vi "HEWH RLT Draw Tester.vi"(8 "Error In":errorcluster) -> (0 "Error Out":errorcluster)   [LabVIEW 2016]
uses:
  Utility/Type Definitions/UTILITY Notifier.ctl
  Utility/Save File/File Setup.lvlib
  Utility/Save File/File Setup (Public)/Type Definition/Save File DOE Configuration State.ctl
  Type Definitions/HEWH Valve Bank Positions.ctl
  Custom Instrument Control/MW100/Type Definitions/HEWH MW100 Channel Numbers.ctl
  Utility/LabVIEW GEA2 Toolkit v1.0.0.0/library/GEA2_Toolkit.lvlib
  Utility/Custom Pallet Controls/Custom Pallet DBL.ctl
  Type Definitions/HEWH Power Elements.ctl
  Type Definitions/HEWH Draw Pattern Setup.ctl
  Type Definitions/HEWH Termination Condition Cluster.ctl
  Type Definitions/HEWH Power Data.ctl
  Utility/Type Definitions/UTILITY Power Analyzer.ctl
  Type Definitions/HEWH Output Information.ctl
  Type Definitions/HEWH Tank Indicator.ctl
  Utility/Custom Pallet Controls/Custom Pallet Timer.ctl
  Type Definitions/HEWH RLT Cycle Conditions.ctl
  Utility/Type Definitions/UTILITY Power Inputs Control.ctl
  Drivers/IND560 Scale Monitor/Type Definitions/IND560 Configuration.ctl
  Type Definitions/HEWH Agilent Cluster.ctl
  Utility/Type Definitions/UTILITY TC Coefficients.ctl
  Washer DOE/Type Definitions/DOE Test Fixture Hardware.ctl
  Washer DOE/Configuration/GEA2.ctl
  Washer DOE/Type Definitions/DOE Capacity Measurments.ctl
  <vilib>/Platform/fileVersionInfo.llb/FileVersionInformation.ctl
  Utility/Custom Pallet Controls/Custom Pallet String.ctl
  Utility/Save File/File Setup (Public)/Type Definition/Save File DISH Dishwasher Details.ctl
  Washer DOE/Type Definitions/DOE Main Control.ctl
  Utility/Save File/File Setup (Public)/Type Definition/Save File DOE Data Save Filepaths.ctl
  Utility/Save File/File Setup (Public)/Type Definition/Save File DOE File Path Control.ctl
  Utility/Save File/File Setup (Public)/Type Definition/Save File DOE LabView Program.ctl
  Custom Instrument Control/MW100/Type Definitions/Station ID Selector.ctl
  Utility/Save File/File Setup (Public)/Type Definition/Save File HEWH Heating Control Mode.ctl
  Type Definitions/PRAT Test.ctl
  Type Definitions/HEWH Calc and Calibration.ctl
  Support VIs/Draw Water Specific/Type Definitions/Terminate Draw Conditions.ctl
  Type Definitions/HEWH Start Conditions.ctl
  Type Definitions/HEWH Specific DAQ.ctl
  Utility/Save File/Public/Type Definitions/Save File Unit Type.ctl
  Utility/Save File/Save File.lvlib
  Utility/Save File/Public/Type Definitions/Save File Appliance Display.ctl
  Utility/Save File/Public/Type Definitions/Save File Washer.ctl
  Support VIs/Draw Water Specific/Type Definitions/Check Special Condtions.ctl
  Type Definitions/HEWH Draw Flag ENUM.ctl
  Support VIs/Draw Water Specific/Type Definitions/HEWH Special Condition Check.ctl
  Drivers/Omega FMA-1600A Series Gas Flow Meter/Type Definitions/FMA1600A COM Ports.ctl
  Washer DOE/Type Definitions/DOE Appliance Common.ctl
  Washer DOE/Type Definitions/DOE Dryer Standard.ctl
  Utility/Save File/File Setup (Public)/Type Definition/DPT IMC Data.ctl
panel:
  out "Numeric":i32
  in  "Retry Count":i32=5
  out "MW100":refnum<visa-resource-name>
  out "Main Loop Rate":dbl format="%0.2f"
  out "File  Version":string="Parametric Stand"
  in  "Filepath Output":T1={"General Setup Paths"={"Calibration File Path"=path "C:/Program Files/GE/Washer DOE/CalibrationDates.txt", "DOE Capacity Path"=path "C:/Program Files/GE/Washer DOE/DOE Capacity.txt", "Data Folder Path"=path "C:/Program Files/GE/Washer DOE/CalibrationDates.txt", "RLT Backup Data Path"=path "C:/Program Files/GE/Washer DOE/CalibrationDates.txt", "Tool Base Path"=path "C:/Program Files/GE/Washer DOE/CalibrationDates.txt", "General Startup Config Path"=path "C:/Program Files/GE/Washer DOE/CalibrationDates.txt", "File Save Previous Run Path"=path "C:/Program Files/GE/Washer DOE/CalibrationDates.txt", "File Save Configuration Data Path"=path "C:/Program Files/GE/Washer DOE/CalibrationDates.txt"}, "Data File Paths"={"Data File Path"=path "", "Debug File Path"=path "", "Bus Log Path"=path "", "Current"=path "", "Summary"=path ""}, "New Summary Created"=FALSE, "Check Location Interval (Second)"=0}
  in  "Washer Controls":T3={"Test Fixture Hardware"={"Power "={"Yokogawa"={"WT210"={"Sample Rate (1: 0.25s)"=1, "A Range (12: 20A)"=12, "V Range (6: 600V)"=4, "Power VISA Yokogawa WT210"="WT210"}, "WT500"={"Power VISA Yokogawa WT500"="WT500", "V Range (8: 1000V)"=0, "I Range (7: 40A)"=0, "Update Rate (3: 500ms)"=2}, "WT310_2"={"Sample Rate (1: 0.25s)"=60, "A Range (12: 20A)"=11, "V Range (6: 600V)"=4, "Power VISA Yokogawa WT310_2"="WT310_2"}, "WT310_3"={"Sample Rate (1: 0.25s)"=1, "A Range (12: 20A)"=11, "V Range (6: 600V)"=4, "Power VISA Yokogawa WT310_3"="WT310_3"}}, "Aplus"={"Aplus IP Address"="192.168.1.101", "Remote Port"=502, "Instrument"="APLUS", "Instr Driver Revision"="1.03.0053"}, "Power Limits"={"Crest Factor"={"Upper Limit"=1.49, "Lower Limit"=1.34}, "Harmonic Content"={"Uthd"=2.0}, "Voltage"={"% Error"=2.0}, "Stability"={"<1 Watt "={"Wattage"=1.0, "Slope (mW/H)"=10.0}, ">1 Watt"={"1%Power/Hour"=1.0}}}, "Nominal Voltage"=120, "Time Limit (s)"=10800.0, "Power Variation Limit (%)"=50.0, "Power Supply"={"Chroma 61605"="CHROMA", "Use Chroma?"=FALSE}}, "Weight Scale"={"Com Options"={"IND560Scale VISA"="LaurelMeter_Hot", "IP Address"="192.168.1.50", "Remote Port"=502, "Setra Scale VISA"="SETRA", "GSE 350"="GSE350"}, "Select Scale"=""}, "Flow Rates"={"Laurel Cold IP Address"="", "Laurel Hot IP Address"="", "Hot Water Laurel VISA"="34972A_3", "Cold Water Laurel VISA"="MW100", "Remote Port"=0, "Laurel Communication Type"="", "Meters To Collect (Hot Cold)"="", "HOT Laurel Reference"=refnum, "COLD Laurel Reference"=refnum}, "Analog Data"={"Agilent"={"Agilent 34972_1"="34972A_1", "Agilent 34972_2"="34972A_2", "Agilent 34972_3"="34972A_3", "Agilent 34972_4"="34972A_3", "Agilent 34972_5"="34972A_3", "Agilent 34972_6"="34972A_3", "Agilent Gain"=0.0, "TC Type (K,J,T)"="", "Instrument IDN?"="", "TC Channels-List"="", "Analog Channels-List"="", "Agilent Cluster Array"=[], "TC Channels-List 2"="", "Analog Channels-List 2"=""}, "Yokogawa"={"MW100"="MW100", "Intellifaucet"=FALSE}, "Select Analog"="", "TC Coefficients"={"TC Coefficients 1"=[], "TC Coefficients 2"=[], "TC Coefficients 3"=[], "TC Coefficients 4"=[], "TC Coefficients 5"=[], "TC Coefficients 6"=[], "TC Coefficients 7"=[]}, "NI Tasks (Dryer DOE)"=["TC Temps-Module 1", "TC Temps-Module 2", "TC Temps-Module 3", "TC Temps-Module 4", "TC Temps-Module 5", "Gas and Temp-Module 6", "AC_DC Events-Module 7"], "Laurel Analog"={"Laurel IP (Water Temp)"="", "Laurel IP (Pressure)"=""}}, "ITHX-Temp Humidity"={"IP Address 1"="", "Remote Port"=0, "IP Address 2"="", "IP Address 3"=""}, "Gas Meter COM Ports"={"Gas Meter 1"="COM3", "Gas Meter 2"="COM4", "Gas Meter 3"="COM5", "Gas Meter 4"="COM6", "Gas Meter 5"="COM7", "Gas Meter 6"="COM8"}, "Barometric Pressure"={"HEISE 901A"="HEISE", "Use Barometer?"=FALSE}}, "GEA2"={"Address"=35, "Source"=228, "Viper/Hawk"=0}, "DOE Capacity Measurments"={"Weight 1"=35.0, "Model Number 1"="", "Temp 1"=0.0, "Serial Number 1"="", "Lab Number 1"="", "Lab Number 2"="", "Serial Number 2"="", "Temp 2"=0.0, "Model Number 2"="", "Weight 2"=0.0, "Lab Number 3"="", "Serial Number 3"="", "Temp 3"=0.0, "Model Number 3"="", "Weight 3"=0.0, "Lab Number 4"="", "Serial Number 4"="", "Temp 4"=0.0, "Model Number 4"="", "Weight 4"=0.0, "Capacity Measurment Output String"=[]}, "Initialize.Washer In"={"Appliance Details"={"FileVersionInfo"={"FileVersion"="", "ProductName"="", "InternalName"="", "CompanyName"="", "LegalCopyright"="", "FileDescription"=""}, "Dishwasher Info"={"Open Cup Weight (gm):"=0.0, "Auto Cup Weight (gm):"=0.0, "Detergent-Dish:"="", "Inlet Temperature-Dish:"="", "Cycle Mode-Dish:"="", "Unit Control-Dish:"="", "Manufacturer-Dish:"=""}, "Washer Info"={"Hot Water Temperature (Fahrenheit):"="", "Cold Water Temperature (Fahrenheit):"="", "Capacity (cu.ft):"=0.0, "Initial Cloth Weight:"=0.0, "Cloth Lot:"=60, "Model Family:"="", "Program Name:"="", "Cycle Selection:"="", "Wash Temperature:"="", "Rinse Temperature:"="", "Load Size:"=""}, "File Name Output Array"=[], "Calibration Output Array"=[], "Appliance Common"={"Engineer:"="", "Model Number:"="", "Serial Number:"="", "Comments:"="", "Station ID:"="", "Technician:"="", "TR Number:"="", "Lab ID:"="", "Voltage:"="", "Water Pressure (PSI):"="", "Test Date:"="", "Computer Name:"="", "IP Address:"="", "Ambient RH:"="", "Frequency:"="", "Build:"="", "Filename:"="", "Test Type:"="", "Load Run #:"=17, "Ambient Temperature (F):"="", "File Path:"=path "", "Cycles Per Year"=0}, "Water Heater"={"Heating Mode:"=""}, "Dryer"={"Heat Setting:"="", "Washer Water Temperature (60 ± 5°F):"=7, "Water Hardness (PPM):"=7, "Dryness Setting:"="", "Dryer Type:"="", "Exhaust:"="", "Drying Cycle:"="", "Load Type:"="", "Nominal Load Weight"="", "Dryer Initial IMC Data"={"Measured IMC (lbs)"=100.0, "Actual Initial RMC (%)"=7.0, "RMC (Desired %)"=5.0, "Bone Dry Wt(lbs)"=60.0, "Tolerance(%)"=5.0, "Actual Final RMC (%)"=7.0, "CEF (lbf/kWh)"=0.0, "Minimum Weight (lbf)"=0.0, "Average Weight (lbf)"=0.0, "Maximum Weight (lbf)"=0.0, "Measured IMC In Range?"=FALSE, "Moisture Reduction Factor"=55.5, "Field Use Factor"=1.04, "Empty Dryer Cold Weigth"=0.0, "Energy Standard"=enum."D2-Automatic Dryer", "Weight Cloth (lbs)"=0.0, "Relative Moisture Content (%)"=0.0, "Relative Moisture Content - Avg (%)"=0.0}}}, "Display Data (RLT)"={"Status Color"=0, "Serial Number Display"="", "Cycle Count Display"=0, "Station Label Display"="", "Current Run Start Time Display"=0.0, "Board ID Display"="", "RPM Display"=0, "Current Display"=0.0, "Current Path Display"=path "", "Saving Display"=FALSE, "Unit Type Display"=enum."", "Total Time On Display"=0.0, "UI Button"=FALSE}}} {"Initialize.Washer In"."Display Data (RLT)"."Current Display" format="%.2f"; "Initialize.Washer In"."Display Data (RLT)"."Cycle Count Display" format="%04d"; "Initialize.Washer In"."Appliance Details"."Dryer"."Dryer Initial IMC Data"."Maximum Weight (lbf)" format="%03_6g"; "Initialize.Washer In"."Appliance Details"."Dryer"."Dryer Initial IMC Data"."Average Weight (lbf)" format="%03_6g"; "Initialize.Washer In"."Appliance Details"."Dryer"."Dryer Initial IMC Data"."Minimum Weight (lbf)" format="%03_6g"; "Initialize.Washer In"."Appliance Details"."Dryer"."Dryer Initial IMC Data"."CEF (lbf/kWh)" format="%03_6g"; "Initialize.Washer In"."Appliance Details"."Dryer"."Dryer Initial IMC Data"."Actual Final RMC (%)" format="%03_6g"; "Initialize.Washer In"."Appliance Details"."Dryer"."Dryer Initial IMC Data"."Tolerance(%)" format="%0#_6g"; "Initialize.Washer In"."Appliance Details"."Dryer"."Dryer Initial IMC Data"."Bone Dry Wt(lbs)" format="%03_6g"; "Initialize.Washer In"."Appliance Details"."Dryer"."Dryer Initial IMC Data"."RMC (Desired %)" format="%0#_6g"; "Initialize.Washer In"."Appliance Details"."Dryer"."Dryer Initial IMC Data"."Actual Initial RMC (%)" format="%03_6g"; "Initialize.Washer In"."Appliance Details"."Dryer"."Dryer Initial IMC Data"."Measured IMC (lbs)" format="%0#_6g"; "GEA2"."Address" format="%x"; "GEA2"."Source" format="%x"; "GEA2"."Viper/Hawk" items=["Viper", "Hawk"]; "Test Fixture Hardware"."Power"."Yokogawa"."WT310_3"."V Range (6: 600V)" items=["Auto", "15V", "30V", "60V", "150V", "300V", "600V"]; "Test Fixture Hardware"."Power"."Yokogawa"."WT310_3"."A Range (12: 20A)" items=["Auto", "5mA", "10mA", "20mA", "50mA", "100mA", "200mA", "0.5A", "1A", "2A", "5A", "10A", "20A", "50mV", "100mV", "200mV", "2.5V", "5V", "10V"]; "Test Fixture Hardware"."Power"."Yokogawa"."WT310_3"."Sample Rate (1: 0.25s)" items=["0.1s", "0.25s", "0.5s", "1s", "2s", "5s"]; "Test Fixture Hardware"."Power"."Yokogawa"."WT310_2"."V Range (6: 600V)" items=["Auto", "15V", "30V", "60V", "150V", "300V", "600V"]; "Test Fixture Hardware"."Power"."Yokogawa"."WT310_2"."A Range (12: 20A)" items=["Auto", "5mA", "10mA", "20mA", "50mA", "100mA", "200mA", "0.5A", "1A", "2A", "5A", "10A", "20A", "50mV", "100mV", "200mV", "2.5V", "5V", "10V"]; "Test Fixture Hardware"."Power"."Yokogawa"."WT310_2"."Sample Rate (1: 0.25s)" items=["0.1s", "0.25s", "0.5s", "1s", "2s", "5s"]; "Test Fixture Hardware"."Power"."Yokogawa"."WT500"."Update Rate (3: 500ms)" items=["-", "100ms", "200ms", "500ms", "1s", "2s", "5s"]; "Test Fixture Hardware"."Power"."Yokogawa"."WT500"."I Range (7: 40A)" items=["AUTO", "500 mA", "1 A", "2 A", "5 A", "10 A", "20 A", "40 A", "S-AUTO", "50 mV", "100 mV", "200 mV", "500 mV", "1 V", "2 V", "5 V", "10 V", "250 mA", "500 mA", "1 A", "2.5 A", "5 A", "10 A", "20 A", "25 mV", "50 mV", "100 mV", "250 mV", "500 mV", "1 V", "2.5 V", "5 V"]; "Test Fixture Hardware"."Power"."Yokogawa"."WT500"."V Range (8: 1000V)" items=["AUTO", "15", "30", "60", "100", "150", "300", "600", "1000", "7.5", "15", "30", "50", "75", "150", "300", "500"]; "Test Fixture Hardware"."Power"."Yokogawa"."WT210"."V Range (6: 600V)" items=["Auto", "15V", "30V", "60V", "150V", "300V", "600V"]; "Test Fixture Hardware"."Power"."Yokogawa"."WT210"."A Range (12: 20A)" items=["Auto", "5mA", "10mA", "20mA", "50mA", "100mA", "200mA", "0.5A", "1A", "2A", "5A", "10A", "20A", "50mV", "100mV", "200mV", "2.5V", "5V", "10V"]; "Test Fixture Hardware"."Power"."Yokogawa"."WT210"."Sample Rate (1: 0.25s)" items=["0.1s", "0.25s", "0.5s", "1s", "2s", "5s"]}
  out "JKI Loop":i32
  out "Draw Loop":i32
  in  "Debug":bool
  out "States":string[](array[string])
  in  "Tab Control 2":enum32{"Setup", "Graph"}(tab)
  in  "Condition Cluster Output":T21={"Condition #1"=TRUE, "Condition #2"=FALSE, "Special Last Draw (HU Test)"=FALSE, "RTD Out Temperature <="=0.0, "Condition #3"=FALSE, "Mean Tank Temperature <="=0.0, "Condition #4"=FALSE, "Decrease Outlet Temperature \nBy (RTD Out)"=0.0, "Condition #5"=FALSE, "Condition #6"=FALSE, "Time (Seconds)"=0.0, "Condition #7"=FALSE, "Condition #8"=FALSE, "Draw Until Condition"={"UE"=FALSE, "LE"=FALSE, "COMP"=FALSE, "FANS"=FALSE}, "Condition #9"=FALSE}
  in  "Clear Graph Data":bool
  out "XY Graph":T23(graph)
  in  "Pause Graph":bool
  in  "X-Axis":string(combo)
  in  "Y-Axis-1":string(combo)
  in  "Y-Axis-2":string(combo)
  in  "HEWH Power":bool
  out "DAQ Data":T24={"HEWH Standard"={"Voltage (Volts)"=240.0, "Current (Amps)"=0.017575, "Power (Watts)"=4.218, "WattHours (Wh)"=19682.0, "TC Tree (AVG)"=0.0, "Flow Rate (GPM)"=0.0, "Gallons (Gal)"=0.0, "RTD Out (Deg F)"=0.0, "RTD In (Deg F)"=0.0, "RTD Amb (Deg F)"=0.0, "TC Down"=0.0, "UE Event Lead"=0, "LE Event Lead"=0, "TC Tree Array"=[]}, "PRAT"={"Power (Watts) A"=4192.0, "Power (Watts) B"=4192.0, "Power (Watts) C"=4192.0, "Power (Watts) D"=4192.0, "TC1"=0.0, "TC2"=0.0, "TC3"=0.0, "TC4"=0.0, "WattHours (Wh) A"=4192.0, "WattHours (Wh) B"=4192.0, "WattHours (Wh) C"=4192.0, "WattHours (Wh) D"=4192.0, "Ambient"=0.0, "Extra Temp"=0.0}, "Additional Power Data"={"Vthd"=236.2, "Frequency (Hz)"=236.2, "Apparent Power (VA)"=236.2, "Power Factor"=236.2, "Current Crest Factor"=236.2, "Voltage Crest Factor"=236.2, "Integration Time (sec)"=236.2}}
  out "Shutdown":bool=TRUE
  out "Delay Between Draws":T25 format="%<%H:%M:%S>t"
  out "Draw Complete":bool
  out "Timer Reset":bool
  out "Elapsed Time":T25 format="%<%H:%M:%S>t"
  in  "Tab Control":enum32{"Standard", "Custom"}(tab)
  out "Draw Count":i32
  in  "Cycle Condition":T26=enum."Time Delay (Seconds)"
  in  "Delay Between\nDraws (seconds)":dbl=60.0
  in  "Gallon Target":T27=6.0 format="%.2f"
  in  "Purge Time (Seconds)":T27=100.0 format="%.2f"
  in  "GPM Target":T27=3.0 format="%.2f"
  in  "Temperature":T27=58.0 format="%.2f"
  out "Set Status":T22
  out "MW100 Data":string[][](array[string])
  out "Tank Display":T28 {"TC6" format="%.2g"; "TIN" format="%.2g"; "TOUT" format="%.2g"; "TC5" format="%.2g"; "TC4" format="%.2g"; "TC3" format="%.2g"; "TC2" format="%.2g"; "TC1" format="%.2g"}
  in  "Reset Gallons":bool
  in  "Disable ERD A":bool
  in  "Use EMV List":bool=TRUE
  in  "Start UI Loop":bool=TRUE
  in  "Pressurize Tank":bool=TRUE
  in  "Stop Custom Draw":bool
  in  "Skip Draw":bool
  in  "Skip Purge":bool
  in  "Start Draw Override":bool
  in  "Start Test":bool
  out "Start Draw":bool
  out "Stop Draw Status":bool
  out "Pressurize Tank Status":bool
  out "UI Loop Status":bool
  out "Core HEWH Data out":T29={"Scan Rate Adjust"=0.0, "Draw Count"=0, "Test Patten Setup"={"Total Gallons Schedule"=[], "PRAT/RLT Sequence"=[{"Sequence #"=1.0, "Cycles"=35, "Mode Setting"="", "Flow Rate (GPM)"=0.0, "Temperature (F)"=0.0, "Reset Timer"=FALSE, "Use Temp Decline Method"=FALSE, "Terminate Condition"=enum."C1-Terminate Draw @ Gallon Mark", "Condition Value #1"=1.0, "UE"=FALSE, "LE"=FALSE, "Comp"=FALSE, "Fan"=FALSE, "Test End Time (Sec)"=0.0, "Purge Until Cutout"=FALSE, "Start Conditions"=enum."Heat Source Cutout", "Condition Value #2"=0.0, "Remove Power"=FALSE, "Time"=0.0, "Check Special Cond."=enum."SC1-Do Nothing", "Condition#"=enum."C1", "Draw Flags"=enum."N/A", "Data Processing Delay (FHD 15sec, UEF 5 Sec)"=0.0, "Test Complete"=FALSE}, {"Sequence #"=2.0, "Cycles"=15, "Mode Setting"="", "Flow Rate (GPM)"=0.0, "Temperature (F)"=0.0, "Reset Timer"=FALSE, "Use Temp Decline Method"=FALSE, "Terminate Condition"=enum."C1-Terminate Draw @ Gallon Mark", "Condition Value #1"=1.0, "UE"=FALSE, "LE"=FALSE, "Comp"=FALSE, "Fan"=FALSE, "Test End Time (Sec)"=0.0, "Purge Until Cutout"=FALSE, "Start Conditions"=enum."Heat Source Cutout", "Condition Value #2"=0.0, "Remove Power"=FALSE, "Time"=0.0, "Check Special Cond."=enum."SC1-Do Nothing", "Condition#"=enum."C1", "Draw Flags"=enum."N/A", "Data Processing Delay (FHD 15sec, UEF 5 Sec)"=0.0, "Test Complete"=FALSE}, {"Sequence #"=3.0, "Cycles"=35, "Mode Setting"="", "Flow Rate (GPM)"=0.0, "Temperature (F)"=0.0, "Reset Timer"=FALSE, "Use Temp Decline Method"=FALSE, "Terminate Condition"=enum."C1-Terminate Draw @ Gallon Mark", "Condition Value #1"=2.0, "UE"=FALSE, "LE"=FALSE, "Comp"=FALSE, "Fan"=FALSE, "Test End Time (Sec)"=0.0, "Purge Until Cutout"=FALSE, "Start Conditions"=enum."Heat Source Cutout", "Condition Value #2"=0.0, "Remove Power"=FALSE, "Time"=0.0, "Check Special Cond."=enum."SC1-Do Nothing", "Condition#"=enum."C1", "Draw Flags"=enum."N/A", "Data Processing Delay (FHD 15sec, UEF 5 Sec)"=0.0, "Test Complete"=FALSE}, {"Sequence #"=4.0, "Cycles"=15, "Mode Setting"="", "Flow Rate (GPM)"=0.0, "Temperature (F)"=0.0, "Reset Timer"=FALSE, "Use Temp Decline Method"=FALSE, "Terminate Condition"=enum."C1-Terminate Draw @ Gallon Mark", "Condition Value #1"=2.0, "UE"=FALSE, "LE"=FALSE, "Comp"=FALSE, "Fan"=FALSE, "Test End Time (Sec)"=0.0, "Purge Until Cutout"=FALSE, "Start Conditions"=enum."Heat Source Cutout", "Condition Value #2"=0.0, "Remove Power"=FALSE, "Time"=0.0, "Check Special Cond."=enum."SC1-Do Nothing", "Condition#"=enum."C1", "Draw Flags"=enum."N/A", "Data Processing Delay (FHD 15sec, UEF 5 Sec)"=0.0, "Test Complete"=FALSE}, {"Sequence #"=5.0, "Cycles"=35, "Mode Setting"="", "Flow Rate (GPM)"=0.0, "Temperature (F)"=0.0, "Reset Timer"=FALSE, "Use Temp Decline Method"=FALSE, "Terminate Condition"=enum."C1-Terminate Draw @ Gallon Mark", "Condition Value #1"=0.0, "UE"=FALSE, "LE"=FALSE, "Comp"=FALSE, "Fan"=FALSE, "Test End Time (Sec)"=0.0, "Purge Until Cutout"=FALSE, "Start Conditions"=enum."Heat Source Cutout", "Condition Value #2"=0.0, "Remove Power"=FALSE, "Time"=0.0, "Check Special Cond."=enum."SC1-Do Nothing", "Condition#"=enum."C1", "Draw Flags"=enum."N/A", "Data Processing Delay (FHD 15sec, UEF 5 Sec)"=0.0, "Test Complete"=FALSE}, {"Sequence #"=6.0, "Cycles"=15, "Mode Setting"="", "Flow Rate (GPM)"=0.0, "Temperature (F)"=0.0, "Reset Timer"=FALSE, "Use Temp Decline Method"=FALSE, "Terminate Condition"=enum."C1-Terminate Draw @ Gallon Mark", "Condition Value #1"=0.0, "UE"=FALSE, "LE"=FALSE, "Comp"=FALSE, "Fan"=FALSE, "Test End Time (Sec)"=0.0, "Purge Until Cutout"=FALSE, "Start Conditions"=enum."Heat Source Cutout", "Condition Value #2"=0.0, "Remove Power"=FALSE, "Time"=0.0, "Check Special Cond."=enum."SC1-Do Nothing", "Condition#"=enum."C1", "Draw Flags"=enum."N/A", "Data Processing Delay (FHD 15sec, UEF 5 Sec)"=0.0, "Test Complete"=FALSE}, {"Sequence #"=7.0, "Cycles"=35, "Mode Setting"="", "Flow Rate (GPM)"=0.0, "Temperature (F)"=0.0, "Reset Timer"=FALSE, "Use Temp Decline Method"=FALSE, "Terminate Condition"=enum."C1-Terminate Draw @ Gallon Mark", "Condition Value #1"=1.0, "UE"=FALSE, "LE"=FALSE, "Comp"=FALSE, "Fan"=FALSE, "Test End Time (Sec)"=0.0, "Purge Until Cutout"=FALSE, "Start Conditions"=enum."Heat Source Cutout", "Condition Value #2"=0.0, "Remove Power"=FALSE, "Time"=0.0, "Check Special Cond."=enum."SC1-Do Nothing", "Condition#"=enum."C1", "Draw Flags"=enum."N/A", "Data Processing Delay (FHD 15sec, UEF 5 Sec)"=0.0, "Test Complete"=FALSE}, {"Sequence #"=8.0, "Cycles"=15, "Mode Setting"="", "Flow Rate (GPM)"=0.0, "Temperature (F)"=0.0, "Reset Timer"=FALSE, "Use Temp Decline Method"=FALSE, "Terminate Condition"=enum."C1-Terminate Draw @ Gallon Mark", "Condition Value #1"=1.0, "UE"=FALSE, "LE"=FALSE, "Comp"=FALSE, "Fan"=FALSE, "Test End Time (Sec)"=0.0, "Purge Until Cutout"=FALSE, "Start Conditions"=enum."Heat Source Cutout", "Condition Value #2"=0.0, "Remove Power"=FALSE, "Time"=0.0, "Check Special Cond."=enum."SC1-Do Nothing", "Condition#"=enum."C1", "Draw Flags"=enum."N/A", "Data Processing Delay (FHD 15sec, UEF 5 Sec)"=0.0, "Test Complete"=FALSE}], "Current Sequence Index"=0}, "HEWH Specific DAQ"={"HEWH Data"={"HEWH Standard"={"Voltage (Volts)"=0.0, "Current (Amps)"=0.0, "Power (Watts)"=0.0, "WattHours (Wh)"=0.0, "TC Tree (AVG)"=0.0, "Flow Rate (GPM)"=0.0, "Gallons (Gal)"=0.0, "RTD Out (Deg F)"=0.0, "RTD In (Deg F)"=0.0, "RTD Amb (Deg F)"=0.0, "TC Down"=0.0, "UE Event Lead"=0, "LE Event Lead"=0, "TC Tree Array"=[]}, "PRAT"={"Power (Watts) A"=4192.0, "Power (Watts) B"=4192.0, "Power (Watts) C"=4192.0, "Power (Watts) D"=4192.0, "TC1"=0.0, "TC2"=0.0, "TC3"=0.0, "TC4"=0.0, "WattHours (Wh) A"=4192.0, "WattHours (Wh) B"=4192.0, "WattHours (Wh) C"=4192.0, "WattHours (Wh) D"=4192.0, "Ambient"=0.0, "Extra Temp"=0.0}, "Additional Power Data"={"Vthd"=236.2, "Frequency (Hz)"=236.2, "Apparent Power (VA)"=236.2, "Power Factor"=236.2, "Current Crest Factor"=236.2, "Voltage Crest Factor"=236.2, "Integration Time (sec)"=236.2}}, "Intellif Valve % Open"=0.0, "Power State"={"UE"=FALSE, "LE"=FALSE, "COMP"=FALSE, "FANS"=FALSE}, "Power Analyzer"=enum.""}, "Test Output Data"={"PreDraw Data Table"=[], "Data Table"=[], "MW100 TC Headers"=[]}, "Calc and Calibration"={"Mean SD Var Max Min Array"=[], "Draw Statistics (DBL)"=[], "Calibration Coefficients DBL"=[], "Start Gallons"=0.0, "Starting Temp Decline"=0.0, "K-Factor (Intellifaucet)"=0.0, "All Draw Stats"=[], "RTD Terminate Value"=0.0}, "Current Draw Time"=0.0, "LV Program"=enum."HEWH", "Station ID"=enum."A", "Current Cond"=enum."N/A", "Test Complete"=FALSE} {"Test Patten Setup"."PRAT/RLT Sequence"."Time" format="%<%H:%M:%S>t"; "Test Patten Setup"."Total Gallons Schedule" format="%.2f"}
  in  "Core HEWH Data Input":T29={"Scan Rate Adjust"=0.0, "Draw Count"=0, "Test Patten Setup"={"Total Gallons Schedule"=[], "PRAT/RLT Sequence"=[{"Sequence #"=1.0, "Cycles"=35, "Mode Setting"="", "Flow Rate (GPM)"=0.0, "Temperature (F)"=0.0, "Reset Timer"=FALSE, "Use Temp Decline Method"=FALSE, "Terminate Condition"=enum."C1-Terminate Draw @ Gallon Mark", "Condition Value #1"=1.0, "UE"=FALSE, "LE"=FALSE, "Comp"=FALSE, "Fan"=FALSE, "Test End Time (Sec)"=0.0, "Purge Until Cutout"=FALSE, "Start Conditions"=enum."Heat Source Cutout", "Condition Value #2"=0.0, "Remove Power"=FALSE, "Time"=0.0, "Check Special Cond."=enum."SC1-Do Nothing", "Condition#"=enum."C1", "Draw Flags"=enum."N/A", "Data Processing Delay (FHD 15sec, UEF 5 Sec)"=0.0, "Test Complete"=FALSE}, {"Sequence #"=2.0, "Cycles"=15, "Mode Setting"="", "Flow Rate (GPM)"=0.0, "Temperature (F)"=0.0, "Reset Timer"=FALSE, "Use Temp Decline Method"=FALSE, "Terminate Condition"=enum."C1-Terminate Draw @ Gallon Mark", "Condition Value #1"=1.0, "UE"=FALSE, "LE"=FALSE, "Comp"=FALSE, "Fan"=FALSE, "Test End Time (Sec)"=0.0, "Purge Until Cutout"=FALSE, "Start Conditions"=enum."Heat Source Cutout", "Condition Value #2"=0.0, "Remove Power"=FALSE, "Time"=0.0, "Check Special Cond."=enum."SC1-Do Nothing", "Condition#"=enum."C1", "Draw Flags"=enum."N/A", "Data Processing Delay (FHD 15sec, UEF 5 Sec)"=0.0, "Test Complete"=FALSE}, {"Sequence #"=3.0, "Cycles"=35, "Mode Setting"="", "Flow Rate (GPM)"=0.0, "Temperature (F)"=0.0, "Reset Timer"=FALSE, "Use Temp Decline Method"=FALSE, "Terminate Condition"=enum."C1-Terminate Draw @ Gallon Mark", "Condition Value #1"=2.0, "UE"=FALSE, "LE"=FALSE, "Comp"=FALSE, "Fan"=FALSE, "Test End Time (Sec)"=0.0, "Purge Until Cutout"=FALSE, "Start Conditions"=enum."Heat Source Cutout", "Condition Value #2"=0.0, "Remove Power"=FALSE, "Time"=0.0, "Check Special Cond."=enum."SC1-Do Nothing", "Condition#"=enum."C1", "Draw Flags"=enum."N/A", "Data Processing Delay (FHD 15sec, UEF 5 Sec)"=0.0, "Test Complete"=FALSE}, {"Sequence #"=4.0, "Cycles"=15, "Mode Setting"="", "Flow Rate (GPM)"=0.0, "Temperature (F)"=0.0, "Reset Timer"=FALSE, "Use Temp Decline Method"=FALSE, "Terminate Condition"=enum."C1-Terminate Draw @ Gallon Mark", "Condition Value #1"=2.0, "UE"=FALSE, "LE"=FALSE, "Comp"=FALSE, "Fan"=FALSE, "Test End Time (Sec)"=0.0, "Purge Until Cutout"=FALSE, "Start Conditions"=enum."Heat Source Cutout", "Condition Value #2"=0.0, "Remove Power"=FALSE, "Time"=0.0, "Check Special Cond."=enum."SC1-Do Nothing", "Condition#"=enum."C1", "Draw Flags"=enum."N/A", "Data Processing Delay (FHD 15sec, UEF 5 Sec)"=0.0, "Test Complete"=FALSE}, {"Sequence #"=5.0, "Cycles"=35, "Mode Setting"="", "Flow Rate (GPM)"=0.0, "Temperature (F)"=0.0, "Reset Timer"=FALSE, "Use Temp Decline Method"=FALSE, "Terminate Condition"=enum."C1-Terminate Draw @ Gallon Mark", "Condition Value #1"=0.0, "UE"=FALSE, "LE"=FALSE, "Comp"=FALSE, "Fan"=FALSE, "Test End Time (Sec)"=0.0, "Purge Until Cutout"=FALSE, "Start Conditions"=enum."Heat Source Cutout", "Condition Value #2"=0.0, "Remove Power"=FALSE, "Time"=0.0, "Check Special Cond."=enum."SC1-Do Nothing", "Condition#"=enum."C1", "Draw Flags"=enum."N/A", "Data Processing Delay (FHD 15sec, UEF 5 Sec)"=0.0, "Test Complete"=FALSE}, {"Sequence #"=6.0, "Cycles"=15, "Mode Setting"="", "Flow Rate (GPM)"=0.0, "Temperature (F)"=0.0, "Reset Timer"=FALSE, "Use Temp Decline Method"=FALSE, "Terminate Condition"=enum."C1-Terminate Draw @ Gallon Mark", "Condition Value #1"=0.0, "UE"=FALSE, "LE"=FALSE, "Comp"=FALSE, "Fan"=FALSE, "Test End Time (Sec)"=0.0, "Purge Until Cutout"=FALSE, "Start Conditions"=enum."Heat Source Cutout", "Condition Value #2"=0.0, "Remove Power"=FALSE, "Time"=0.0, "Check Special Cond."=enum."SC1-Do Nothing", "Condition#"=enum."C1", "Draw Flags"=enum."N/A", "Data Processing Delay (FHD 15sec, UEF 5 Sec)"=0.0, "Test Complete"=FALSE}, {"Sequence #"=7.0, "Cycles"=35, "Mode Setting"="", "Flow Rate (GPM)"=0.0, "Temperature (F)"=0.0, "Reset Timer"=FALSE, "Use Temp Decline Method"=FALSE, "Terminate Condition"=enum."C1-Terminate Draw @ Gallon Mark", "Condition Value #1"=1.0, "UE"=FALSE, "LE"=FALSE, "Comp"=FALSE, "Fan"=FALSE, "Test End Time (Sec)"=0.0, "Purge Until Cutout"=FALSE, "Start Conditions"=enum."Heat Source Cutout", "Condition Value #2"=0.0, "Remove Power"=FALSE, "Time"=0.0, "Check Special Cond."=enum."SC1-Do Nothing", "Condition#"=enum."C1", "Draw Flags"=enum."N/A", "Data Processing Delay (FHD 15sec, UEF 5 Sec)"=0.0, "Test Complete"=FALSE}, {"Sequence #"=8.0, "Cycles"=15, "Mode Setting"="", "Flow Rate (GPM)"=0.0, "Temperature (F)"=0.0, "Reset Timer"=FALSE, "Use Temp Decline Method"=FALSE, "Terminate Condition"=enum."C1-Terminate Draw @ Gallon Mark", "Condition Value #1"=1.0, "UE"=FALSE, "LE"=FALSE, "Comp"=FALSE, "Fan"=FALSE, "Test End Time (Sec)"=0.0, "Purge Until Cutout"=FALSE, "Start Conditions"=enum."Heat Source Cutout", "Condition Value #2"=0.0, "Remove Power"=FALSE, "Time"=0.0, "Check Special Cond."=enum."SC1-Do Nothing", "Condition#"=enum."C1", "Draw Flags"=enum."N/A", "Data Processing Delay (FHD 15sec, UEF 5 Sec)"=0.0, "Test Complete"=FALSE}], "Current Sequence Index"=0}, "HEWH Specific DAQ"={"HEWH Data"={"HEWH Standard"={"Voltage (Volts)"=0.0, "Current (Amps)"=0.0, "Power (Watts)"=0.0, "WattHours (Wh)"=0.0, "TC Tree (AVG)"=0.0, "Flow Rate (GPM)"=0.0, "Gallons (Gal)"=0.0, "RTD Out (Deg F)"=0.0, "RTD In (Deg F)"=0.0, "RTD Amb (Deg F)"=0.0, "TC Down"=0.0, "UE Event Lead"=0, "LE Event Lead"=0, "TC Tree Array"=[]}, "PRAT"={"Power (Watts) A"=4192.0, "Power (Watts) B"=4192.0, "Power (Watts) C"=4192.0, "Power (Watts) D"=4192.0, "TC1"=0.0, "TC2"=0.0, "TC3"=0.0, "TC4"=0.0, "WattHours (Wh) A"=4192.0, "WattHours (Wh) B"=4192.0, "WattHours (Wh) C"=4192.0, "WattHours (Wh) D"=4192.0, "Ambient"=0.0, "Extra Temp"=0.0}, "Additional Power Data"={"Vthd"=236.2, "Frequency (Hz)"=236.2, "Apparent Power (VA)"=236.2, "Power Factor"=236.2, "Current Crest Factor"=236.2, "Voltage Crest Factor"=236.2, "Integration Time (sec)"=236.2}}, "Intellif Valve % Open"=0.0, "Power State"={"UE"=FALSE, "LE"=FALSE, "COMP"=FALSE, "FANS"=FALSE}, "Power Analyzer"=enum.""}, "Test Output Data"={"PreDraw Data Table"=[], "Data Table"=[], "MW100 TC Headers"=[]}, "Calc and Calibration"={"Mean SD Var Max Min Array"=[], "Draw Statistics (DBL)"=[], "Calibration Coefficients DBL"=[], "Start Gallons"=0.0, "Starting Temp Decline"=0.0, "K-Factor (Intellifaucet)"=0.0, "All Draw Stats"=[], "RTD Terminate Value"=0.0}, "Current Draw Time"=0.0, "LV Program"=enum."HEWH", "Station ID"=enum."A", "Current Cond"=enum."N/A", "Test Complete"=FALSE} {"Test Patten Setup"."PRAT/RLT Sequence"."Time" format="%<%H:%M:%S>t"; "Test Patten Setup"."Total Gallons Schedule" format="%.2f"}
  out "Message":string="Purging and Calibrating Intellifaucet for 46 Seconds...."
  # "This was a bridge test software. Do not use"
  # "Select Only One Condition"
  # "Just Draw Water!"
  # "Condition #1"
  # "Draw Until Any Heat Source"
  # "Condition #2"
  # "Start Dispense Pattern"
  # "Draw Until Specific Heat Source"
  # "Condition #3"
  # "Dispense PRAT Sequence"
  # "Not Working"
  # "Condition #4"
  # "Condition #5"
  # "Condition #6"
  # "Next Cycle\nCondition"
  # "Conditions During Draw"
  # "Draw Pattern Setup (24 Hour)"
  # "Draw Pattern Setup (24 Hour)"
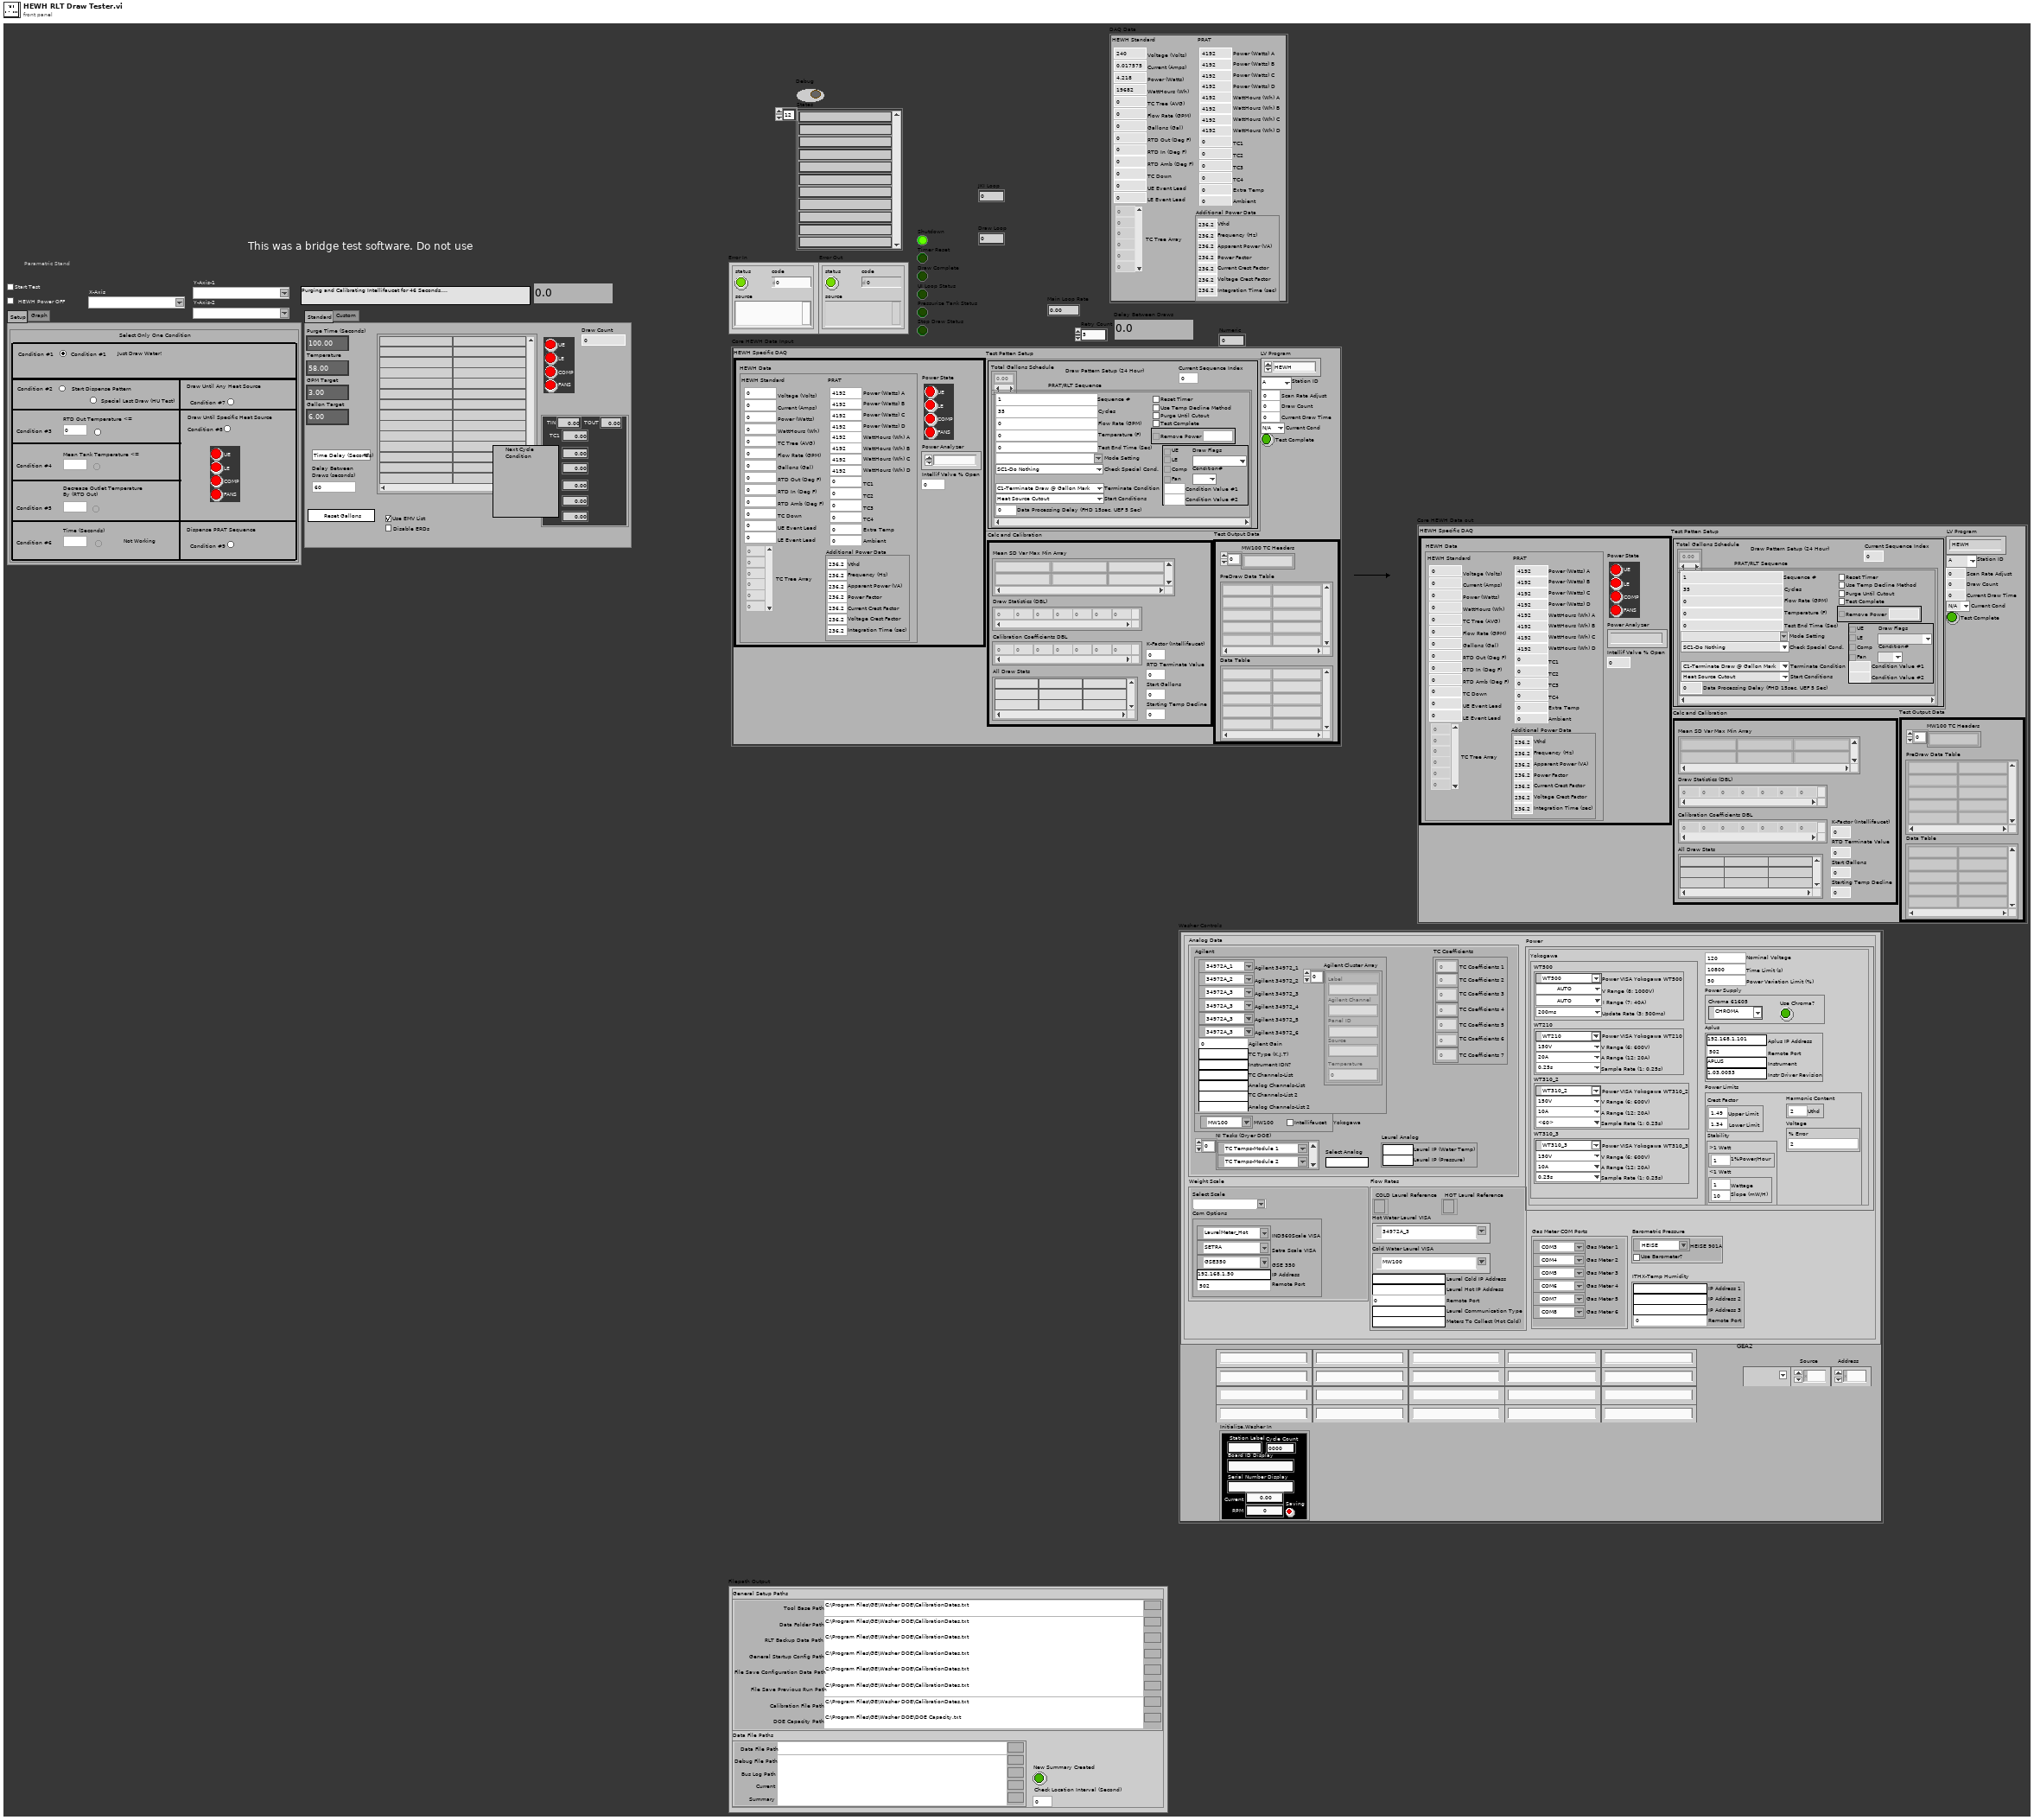
[diagram p1: front panel]
types:
  T1 = typedef "File Setup.lvlib/Save File DOE File Path Control.ctl" = cluster{"General Setup Paths":cluster{"Calibration File Path":path, "DOE Capacity Path":path, "Data Folder Path":path, "RLT Backup Data Path":path, "Tool Base Path":path, "General Startup Config Path":path, "File Save Previous Run Path":path, "File Save Configuration Data Path":path}, "Data File Paths":T2, "New Summary Created":bool, "Check Location Interval (Second)":i32}
  T2 = typedef "File Setup.lvlib/Save File DOE Data Save Filepaths.ctl" = cluster{"Data File Path":path, "Debug File Path":path, "Bus Log Path":path, "Current":path, "Summary":path}
  T3 = typedef "DOE Main Control.ctl" = cluster{"Test Fixture Hardware":T4, "GEA2":T10, "DOE Capacity Measurments":T11, "Initialize.Washer In":T12}
  T4 = typedef "DOE Test Fixture Hardware.ctl" = cluster{"Power ":T5, "Weight Scale":cluster{"Com Options":T6, "Select Scale":string}, "Flow Rates":cluster{"Laurel Cold IP Address":string, "Laurel Hot IP Address":string, "Hot Water Laurel VISA":refnum<visa-resource-name>, "Cold Water Laurel VISA":refnum<visa-resource-name>, "Remote Port":u16, "Laurel Communication Type":string, "Meters To Collect (Hot Cold)":string, "HOT Laurel Reference":refnum<k5>, "COLD Laurel Reference":refnum<k5>}, "Analog Data":cluster{"Agilent":cluster{"Agilent 34972_1":refnum<visa-resource-name>, "Agilent 34972_2":refnum<visa-resource-name>, "Agilent 34972_3":refnum<visa-resource-name>, "Agilent 34972_4":refnum<visa-resource-name>, "Agilent 34972_5":refnum<visa-resource-name>, "Agilent 34972_6":refnum<visa-resource-name>, "Agilent Gain":dbl, "TC Type (K,J,T)":string, "Instrument IDN?":string, "TC Channels-List":string, "Analog Channels-List":string, "Agilent Cluster Array":T7[], "TC Channels-List 2":string, "Analog Channels-List 2":string}, "Yokogawa":cluster{"MW100":refnum<visa-resource-name>, "Intellifaucet":bool}, "Select Analog":string, "TC Coefficients":T8, "NI Tasks (Dryer DOE)":refnum<k21>[], "Laurel Analog":cluster{"Laurel IP (Water Temp)":string, "Laurel IP (Pressure)":string}}, "ITHX-Temp Humidity":cluster{"IP Address 1":string, "Remote Port":u16, "IP Address 2":string, "IP Address 3":string}, "Gas Meter COM Ports":T9, "Barometric Pressure":cluster{"HEISE 901A":refnum<visa-resource-name>, "Use Barometer?":bool}}
  T5 = typedef "UTILITY Power Inputs Control.ctl" = cluster{"Yokogawa":cluster{"WT210":cluster{"Sample Rate (1: 0.25s)":i32, "A Range (12: 20A)":i32, "V Range (6: 600V)":i32, "Power VISA Yokogawa WT210":refnum<visa-resource-name>}, "WT500":cluster{"Power VISA Yokogawa WT500":refnum<visa-resource-name>, "V Range (8: 1000V)":i32, "I Range (7: 40A)":i32, "Update Rate (3: 500ms)":i32}, "WT310_2":cluster{"Sample Rate (1: 0.25s)":i32, "A Range (12: 20A)":i32, "V Range (6: 600V)":i32, "Power VISA Yokogawa WT310_2":refnum<visa-resource-name>}, "WT310_3":cluster{"Sample Rate (1: 0.25s)":i32, "A Range (12: 20A)":i32, "V Range (6: 600V)":i32, "Power VISA Yokogawa WT310_3":refnum<visa-resource-name>}}, "Aplus":cluster{"Aplus IP Address":string, "Remote Port":i32, "Instrument":string, "Instr Driver Revision":string}, "Power Limits":cluster{"Crest Factor":cluster{"Upper Limit":dbl, "Lower Limit":dbl}, "Harmonic Content":cluster{"Uthd":dbl}, "Voltage":cluster{"% Error":dbl}, "Stability":cluster{"<1 Watt ":cluster{"Wattage":dbl, "Slope (mW/H)":dbl}, ">1 Watt":cluster{"1%Power/Hour":dbl}}}, "Nominal Voltage":i32, "Time Limit (s)":dbl, "Power Variation Limit (%)":dbl, "Power Supply":cluster{"Chroma 61605":refnum<visa-resource-name>, "Use Chroma?":bool}}
  T6 = typedef "IND560 Configuration.ctl" = cluster{"IND560Scale VISA":refnum<visa-resource-name>, "IP Address":string, "Remote Port":u16, "Setra Scale VISA":refnum<visa-resource-name>, "GSE 350":refnum<visa-resource-name>}
  T7 = typedef "HEWH Agilent Cluster.ctl" = cluster{"Label":string, "Agilent Channel":string, "Panel ID":string, "Source":string, "Temperature":dbl}
  T8 = typedef "UTILITY TC Coefficients.ctl" = cluster{"TC Coefficients 1":dbl[], "TC Coefficients 2":dbl[], "TC Coefficients 3":dbl[], "TC Coefficients 4":dbl[], "TC Coefficients 5":dbl[], "TC Coefficients 6":dbl[], "TC Coefficients 7":dbl[]}
  T9 = typedef "FMA1600A COM Ports.ctl" = cluster{"Gas Meter 1":refnum<visa-resource-name>, "Gas Meter 2":refnum<visa-resource-name>, "Gas Meter 3":refnum<visa-resource-name>, "Gas Meter 4":refnum<visa-resource-name>, "Gas Meter 5":refnum<visa-resource-name>, "Gas Meter 6":refnum<visa-resource-name>}
  T10 = typedef "GEA2.ctl" = cluster{"Address":u8, "Source":u8, "Viper/Hawk":u8}
  T11 = typedef "DOE Capacity Measurments.ctl" = cluster{"Weight 1":dbl, "Model Number 1":string, "Temp 1":dbl, "Serial Number 1":string, "Lab Number 1":string, "Lab Number 2":string, "Serial Number 2":string, "Temp 2":dbl, "Model Number 2":string, "Weight 2":dbl, "Lab Number 3":string, "Serial Number 3":string, "Temp 3":dbl, "Model Number 3":string, "Weight 3":dbl, "Lab Number 4":string, "Serial Number 4":string, "Temp 4":dbl, "Model Number 4":string, "Weight 4":dbl, "Capacity Measurment Output String":string[][]}
  T12 = typedef "Save File.lvlib/Save File Washer.ctl" = cluster{"Appliance Details":T13, "Display Data (RLT)":T19}
  T13 = typedef "File Setup.lvlib/Save File DISH Dishwasher Details.ctl" = cluster{"FileVersionInfo":T14, "Dishwasher Info":cluster{"Open Cup Weight (gm):":dbl, "Auto Cup Weight (gm):":dbl, "Detergent-Dish:":string, "Inlet Temperature-Dish:":string, "Cycle Mode-Dish:":string, "Unit Control-Dish:":string, "Manufacturer-Dish:":string}, "Washer Info":cluster{"Hot Water Temperature (Fahrenheit):":string, "Cold Water Temperature (Fahrenheit):":string, "Capacity (cu.ft):":dbl, "Initial Cloth Weight:":dbl, "Cloth Lot:":i32, "Model Family:":string, "Program Name:":string, "Cycle Selection:":string, "Wash Temperature:":string, "Rinse Temperature:":string, "Load Size:":string}, "File Name Output Array":string[][], "Calibration Output Array":string[][], "Appliance Common":T15, "Water Heater":cluster{"Heating Mode:":string}, "Dryer":cluster{"Heat Setting:":T16, "Washer Water Temperature (60 ± 5°F):":u16, "Water Hardness (PPM):":u16, "Dryness Setting:":T16, "Dryer Type:":string, "Exhaust:":string, "Drying Cycle:":string, "Load Type:":string, "Nominal Load Weight":string, "Dryer Initial IMC Data":T17}}
  T14 = typedef "FileVersionInformation.ctl" = cluster{"FileVersion":string, "ProductName":string, "InternalName":string, "CompanyName":string, "LegalCopyright":string, "FileDescription":string}
  T15 = typedef "DOE Appliance Common.ctl" = cluster{"Engineer:":string, "Model Number:":string, "Serial Number:":string, "Comments:":string, "Station ID:":string, "Technician:":string, "TR Number:":string, "Lab ID:":string, "Voltage:":string, "Water Pressure (PSI):":string, "Test Date:":string, "Computer Name:":string, "IP Address:":string, "Ambient RH:":string, "Frequency:":string, "Build:":string, "Filename:":string, "Test Type:":string, "Load Run #:":i32, "Ambient Temperature (F):":string, "File Path:":path, "Cycles Per Year":u32}
  T16 = typedef "Custom Pallet String.ctl" = string
  T17 = typedef "DPT IMC Data.ctl" = cluster{"Measured IMC (lbs)":dbl, "Actual Initial RMC (%)":dbl, "RMC (Desired %)":dbl, "Bone Dry Wt(lbs)":dbl, "Tolerance(%)":dbl, "Actual Final RMC (%)":dbl, "CEF (lbf/kWh)":dbl, "Minimum Weight (lbf)":dbl, "Average Weight (lbf)":dbl, "Maximum Weight (lbf)":dbl, "Measured IMC In Range?":bool, "Moisture Reduction Factor":dbl, "Field Use Factor":dbl, "Empty Dryer Cold Weigth":dbl, "Energy Standard":T18, "Weight Cloth (lbs)":dbl, "Relative Moisture Content (%)":dbl, "Relative Moisture Content - Avg (%)":dbl}
  T18 = typedef "DOE Dryer Standard.ctl" = enum16{"D2-Automatic Dryer", "D2-Timer Dryer", "D1-Automatic Dryer", "D1-Timer Dryer", "Other"}
  T19 = typedef "Save File Appliance Display.ctl" = cluster{"Status Color":u32, "Serial Number Display":string, "Cycle Count Display":i32, "Station Label Display":string, "Current Run Start Time Display":dbl, "Board ID Display":string, "RPM Display":u32, "Current Display":dbl, "Current Path Display":path, "Saving Display":bool, "Unit Type Display":T20, "Total Time On Display":dbl, "UI Button":bool}
  T20 = typedef "Save File.lvlib/Save File Unit Type.ctl" = enum32{"", "Viper", "Hawk", "2015"}
  T21 = typedef "HEWH Termination Condition Cluster.ctl" = cluster{"Condition #1":bool, "Condition #2":bool, "Special Last Draw (HU Test)":bool, "RTD Out Temperature <=":dbl, "Condition #3":bool, "Mean Tank Temperature <=":dbl, "Condition #4":bool, "Decrease Outlet Temperature \nBy (RTD Out)":dbl, "Condition #5":bool, "Condition #6":bool, "Time (Seconds)":dbl, "Condition #7":bool, "Condition #8":bool, "Draw Until Condition":T22, "Condition #9":bool}
  T22 = typedef "HEWH Power Elements.ctl" = cluster{"UE":bool, "LE":bool, "COMP":bool, "FANS":bool}
  T23 = cluster{"Time Array Output":dbl[], "Data Array Output":dbl[]}[]
  T24 = typedef "HEWH Power Data.ctl" = cluster{"HEWH Standard":cluster{"Voltage (Volts)":dbl, "Current (Amps)":dbl, "Power (Watts)":dbl, "WattHours (Wh)":dbl, "TC Tree (AVG)":dbl, "Flow Rate (GPM)":dbl, "Gallons (Gal)":dbl, "RTD Out (Deg F)":dbl, "RTD In (Deg F)":dbl, "RTD Amb (Deg F)":dbl, "TC Down":dbl, "UE Event Lead":i32, "LE Event Lead":i32, "TC Tree Array":dbl[]}, "PRAT":cluster{"Power (Watts) A":dbl, "Power (Watts) B":dbl, "Power (Watts) C":dbl, "Power (Watts) D":dbl, "TC1":dbl, "TC2":dbl, "TC3":dbl, "TC4":dbl, "WattHours (Wh) A":dbl, "WattHours (Wh) B":dbl, "WattHours (Wh) C":dbl, "WattHours (Wh) D":dbl, "Ambient":dbl, "Extra Temp":dbl}, "Additional Power Data":cluster{"Vthd":dbl, "Frequency (Hz)":dbl, "Apparent Power (VA)":dbl, "Power Factor":dbl, "Current Crest Factor":dbl, "Voltage Crest Factor":dbl, "Integration Time (sec)":dbl}}
  T25 = typedef "Custom Pallet Timer.ctl" = dbl
  T26 = typedef "HEWH RLT Cycle Conditions.ctl" = enum16{"Manual", "Full Cutout", "Time Delay (Seconds)"}
  T27 = typedef "Custom Pallet DBL.ctl" = dbl
  T28 = typedef "HEWH Tank Indicator.ctl" = cluster{"TC1":dbl, "TC2":dbl, "TC3":dbl, "TC4":dbl, "TC5":dbl, "TIN":dbl, "TOUT":dbl, "TC6":dbl, "TC6-Color":u32, "TC5-Color":u32, "TC4-Color":u32, "TC3-Color":u32, "TC2-Color":u32, "TC1-Color":u32, "RTD-Out":u32, "RTD-In":u32}
  T29 = typedef "HEWH Output Information.ctl" = cluster{"Scan Rate Adjust":dbl, "Draw Count":i32, "Test Patten Setup":T30, "HEWH Specific DAQ":T38, "Test Output Data":cluster{"PreDraw Data Table":string[][], "Data Table":string[][], "MW100 TC Headers":string[]}, "Calc and Calibration":T40, "Current Draw Time":dbl, "LV Program":T41, "Station ID":T42, "Current Cond":T36, "Test Complete":bool}
  T30 = typedef "HEWH Draw Pattern Setup.ctl" = cluster{"Total Gallons Schedule":dbl[], "PRAT/RLT Sequence":T31[], "Current Sequence Index":i32}
  T31 = typedef "PRAT Test.ctl" = cluster{"Sequence #":dbl, "Cycles":i32, "Mode Setting":T32, "Flow Rate (GPM)":dbl, "Temperature (F)":dbl, "Reset Timer":bool, "Use Temp Decline Method":bool, "Terminate Condition":T33, "Condition Value #1":dbl, "UE":bool, "LE":bool, "Comp":bool, "Fan":bool, "Test End Time (Sec)":dbl, "Purge Until Cutout":bool, "Start Conditions":T34, "Condition Value #2":dbl, "Remove Power":bool, "Time":dbl, "Check Special Cond.":T35, "Condition#":T36, "Draw Flags":T37, "Data Processing Delay (FHD 15sec, UEF 5 Sec)":dbl, "Test Complete":bool}
  T32 = typedef "File Setup.lvlib/Save File HEWH Heating Control Mode.ctl" = string
  T33 = typedef "Terminate Draw Conditions.ctl" = enum16{"C1-Terminate Draw @ Gallon Mark", "C2-Special Last Draw (HU Test)", "C3-RTD Out <=", "C4-Mean Tank Temp <=", "C5-Decrease RTD Out (Deg F)", "C6-Time (Seconds)", "C7-Until Any Heat Source", "C8-Specific Heat Source", "C9-Do Nothing"}
  T34 = typedef "HEWH Start Conditions.ctl" = enum16{"Heat Source Cutout", "At Time (Seconds)", "Every X (Seconds)", "T2 >= X° Below Setpoint", "Seconds From Complete", "Wait for LE & Comp Cutout", "Wait for Comp Cutout", "Wait for LE Cutout", "Wait for UE Cutout"}
  T35 = typedef "Check Special Condtions.ctl" = enum16{"SC1-Do Nothing", "SC2-Check Heat Source (On-C2/Off-C1)", "SC3-Check Skip Condition", "SC4-Check Heat Source ON/Fail"}
  T36 = typedef "HEWH Special Condition Check.ctl" = enum16{"N/A", "C1", "C2", "Reset/Fail", "Skip Draw Sequence"}
  T37 = typedef "HEWH Draw Flag ENUM.ctl" = enum16{"N/A", "None(0)", "Sml(1)", "Med(2)", "SmlMed(3)", "Lrg(4)", "SmlLrg(5)", "MedLrg(6)", "SmlMedLrg(7)"}
  T38 = typedef "HEWH Specific DAQ.ctl" = cluster{"HEWH Data":T24, "Intellif Valve % Open":dbl, "Power State":T22, "Power Analyzer":T39}
  T39 = typedef "UTILITY Power Analyzer.ctl" = enum16{"", "APLUS", "WT210", "WT500", "WT300", "OSI", "Debug", "WT230", "WT300_1", "WT300_2"}
  T40 = typedef "HEWH Calc and Calibration.ctl" = cluster{"Mean SD Var Max Min Array":string[][], "Draw Statistics (DBL)":dbl[][], "Calibration Coefficients DBL":dbl[][], "Start Gallons":dbl, "Starting Temp Decline":dbl, "K-Factor (Intellifaucet)":dbl, "All Draw Stats":string[][], "RTD Terminate Value":dbl}
  T41 = typedef "File Setup.lvlib/Save File DOE LabView Program.ctl" = enum16{"No Name Found", "DOE Stand", "Dishwasher Kitchen", "Portable Stand", "HEWH", "Dryer", "Dryer WILT", "HCC", "PRAT", "HEWH RLT"}
  T42 = typedef "Station ID Selector.ctl" = enum16{"", "A", "B", "C", "D", "Global"}
  T43 = typedef "Semaphore RefNum" = refnum<k1>
  T44 = enum32{"invalid app kind", "Development System", "Run Time System", "Student Edition", "Embedded LabVIEW", "Evaluation", "Custom"}
  T45 = typedef "UTILITY Notifier.ctl" = enum16{"Set", "Read", "Release Ref"}
  T46 = typedef "HEWH Valve Bank Positions.ctl" = enum16{"Heating", "Purge", "Resting", "Draw"}
  T47 = enum32{"Invalid", "Standard", "Closed", "Hidden", "Minimized", "Maximized"}
  T48 = typedef "File Setup.lvlib/Save File DOE Configuration State.ctl" = enum16{"Open Front Panel", "Load Config"}
  T49 = typedef "HEWH MW100 Channel Numbers.ctl" = string
  T50 = cluster{"Core":cluster{"Current VI Reference":refnum<vi>, "Close Panel on Exit?":bool}, "Washer Controls":T3, "Filepath Output":T1, "Core HEWH Data Input":T29, "Main Power":bool, "Plot Array":dbl[][], "Total Array":string[][], "Save Data":string[][]}
  T51 = cluster{"Current VI Reference":refnum<vi>, "Close Panel on Exit?":bool}
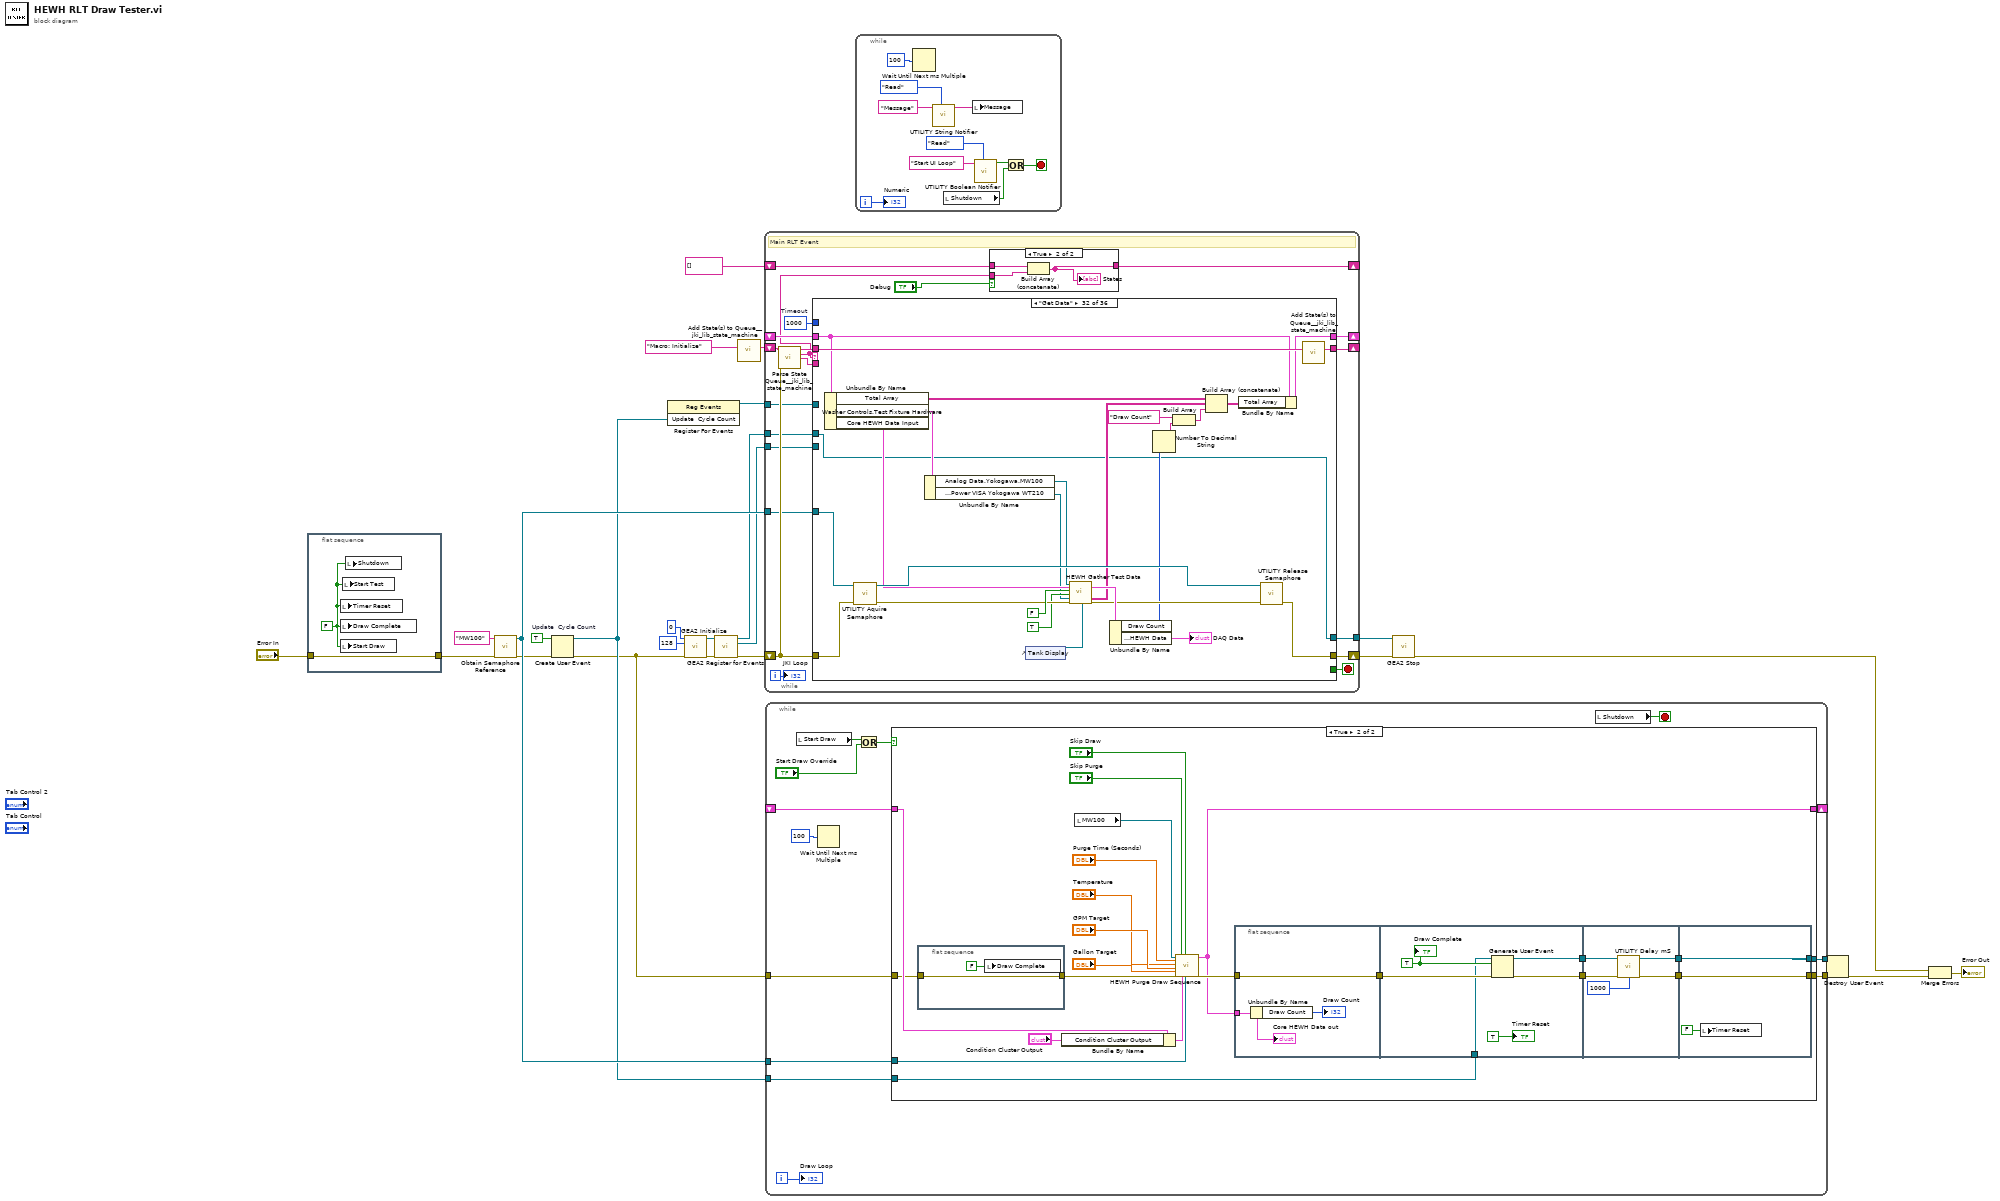
[diagram p0: block diagram]
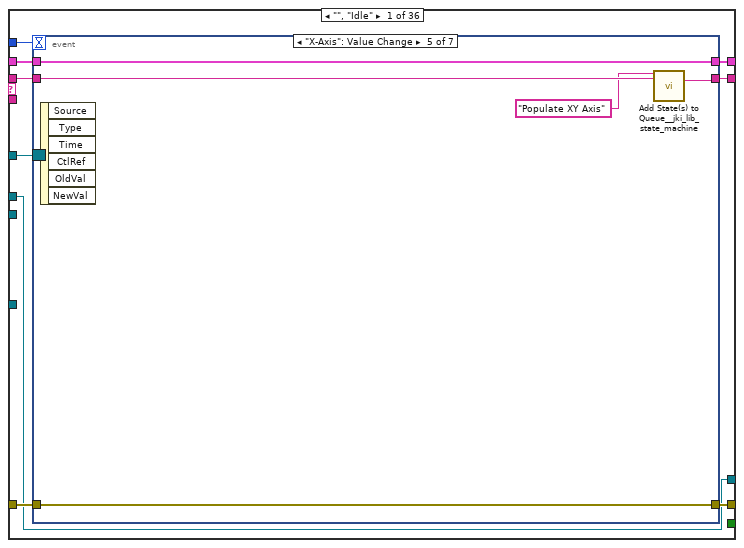
[diagram p3: hidden frame]
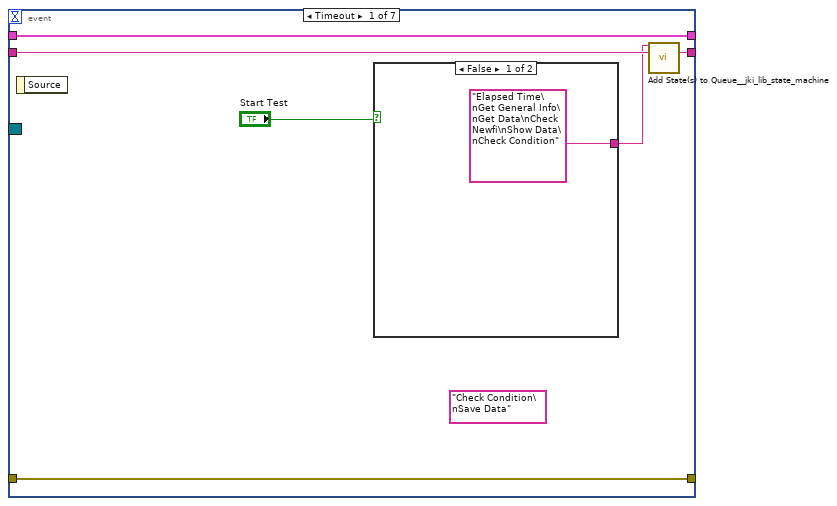
[diagram p4: hidden frame]
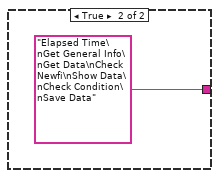
[diagram p5: hidden frame]
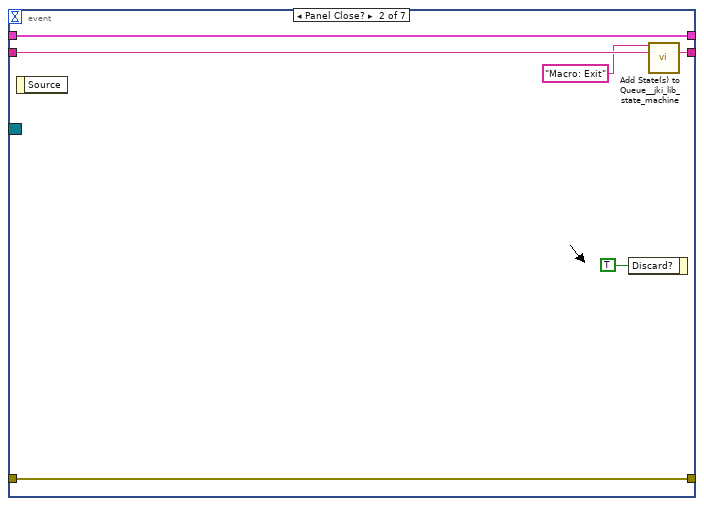
[diagram p6: hidden frame]
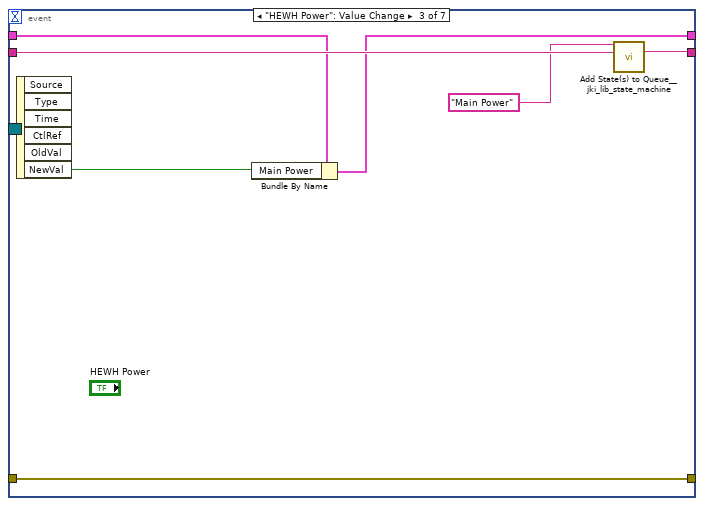
[diagram p7: hidden frame]
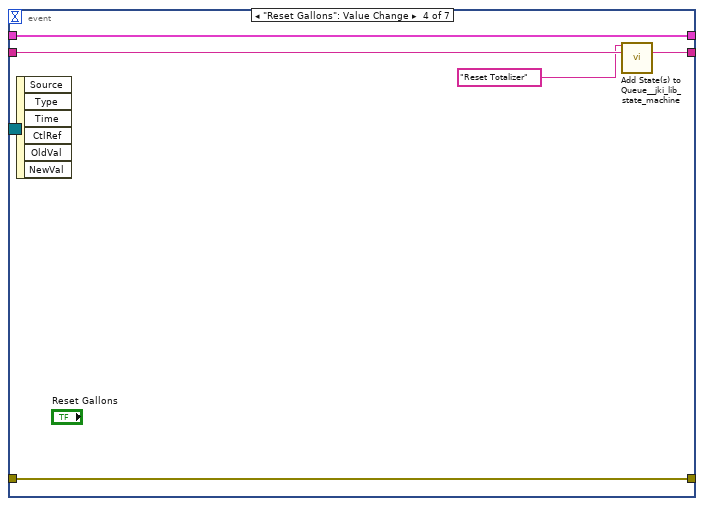
[diagram p8: hidden frame]
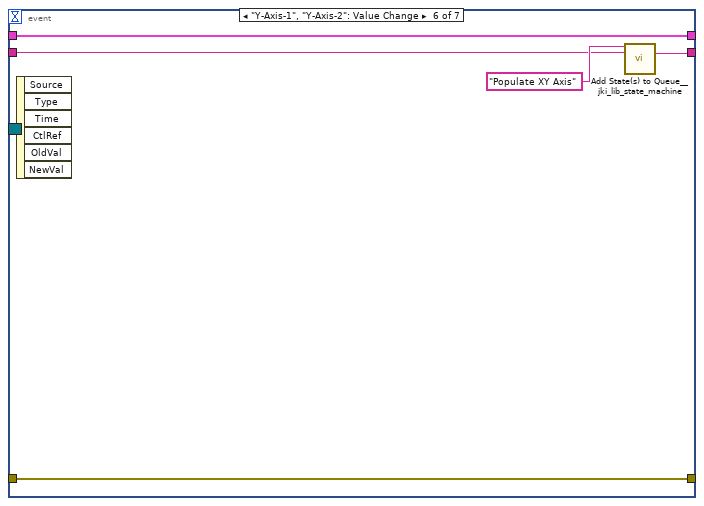
[diagram p9: hidden frame]
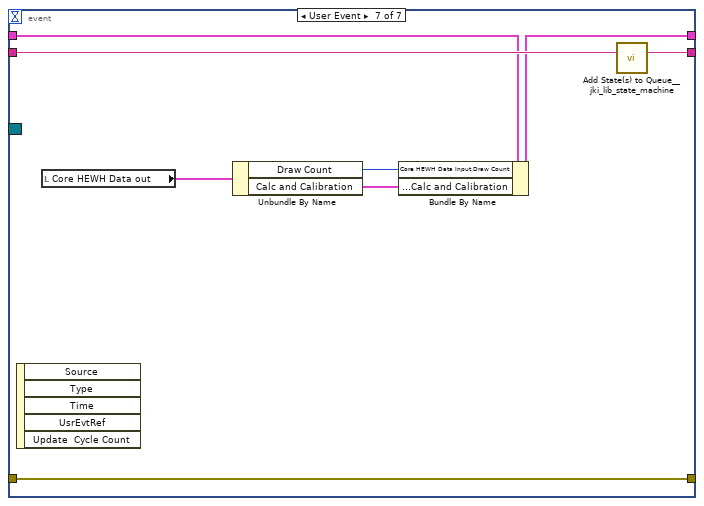
[diagram p10: hidden frame]
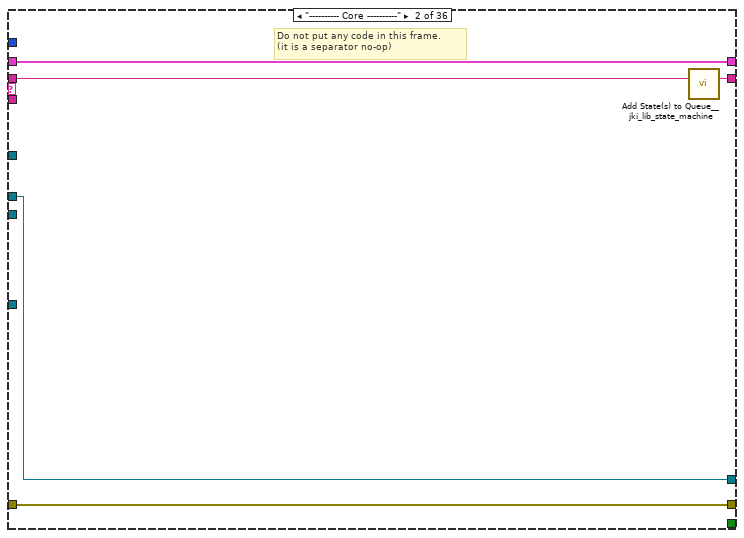
[diagram p11: hidden frame]
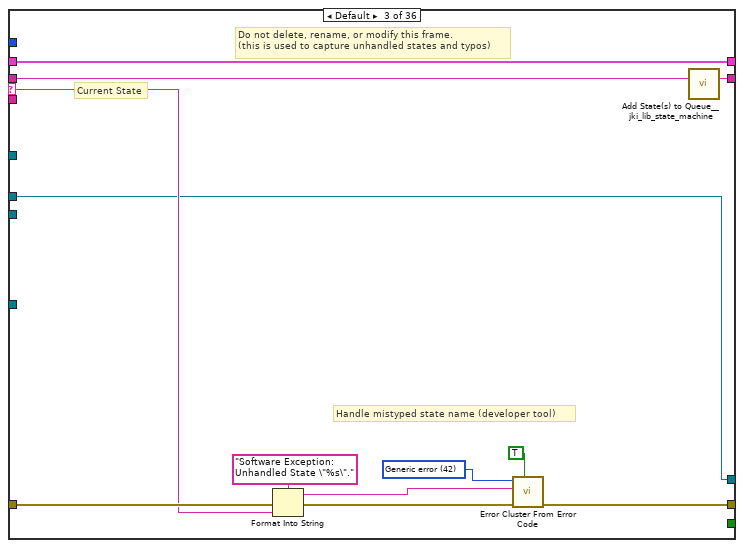
[diagram p12: hidden frame]
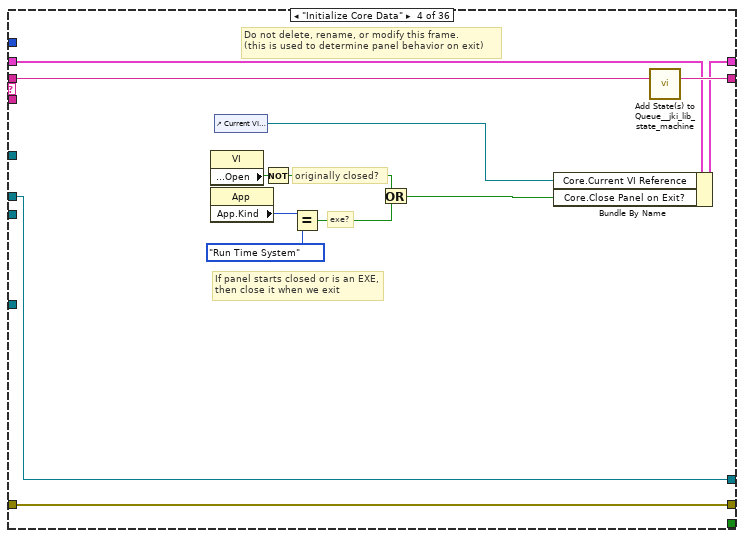
[diagram p13: hidden frame]
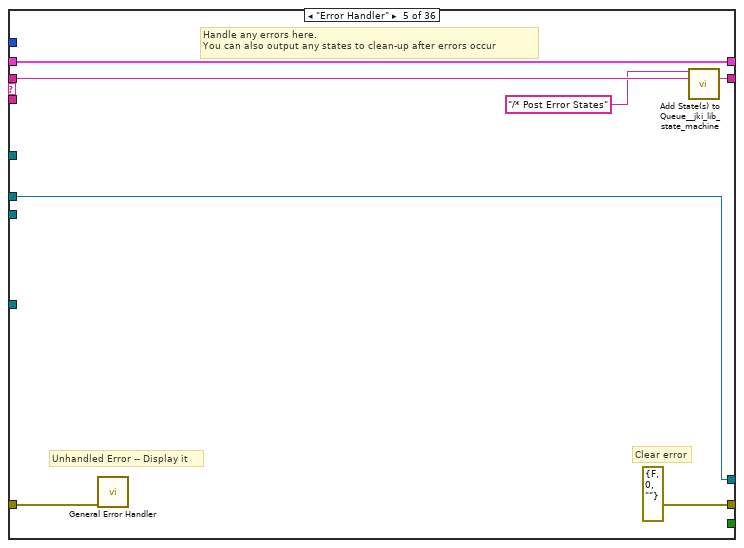
[diagram p14: hidden frame]
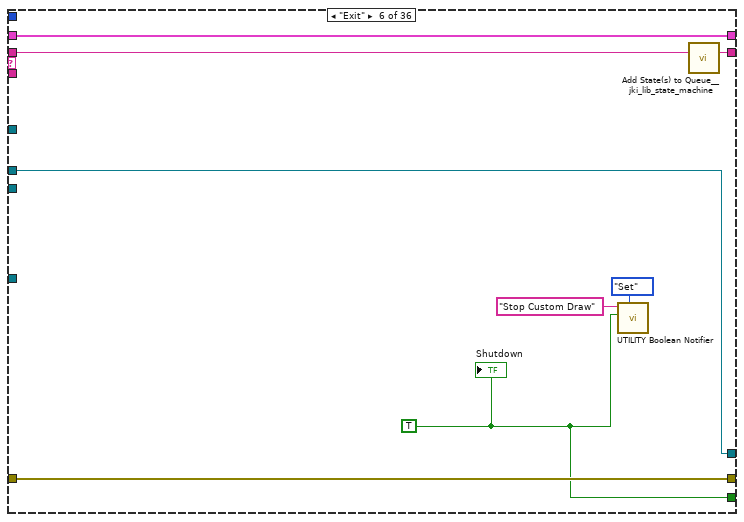
[diagram p15: hidden frame]
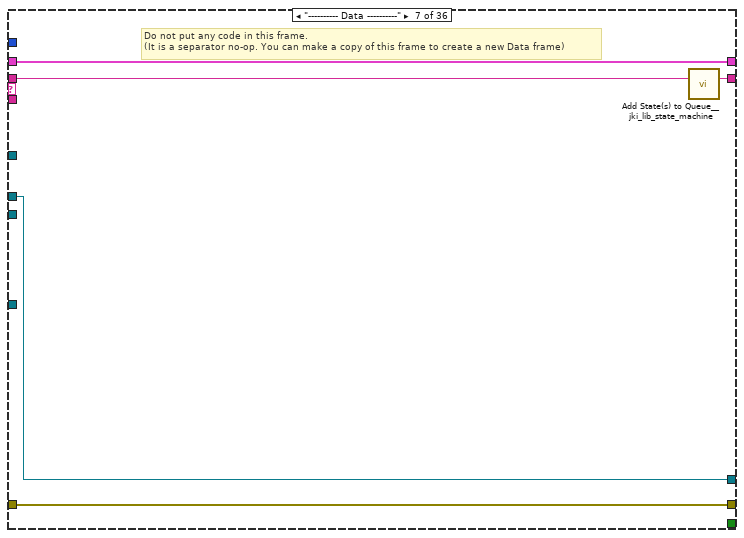
[diagram p16: hidden frame]
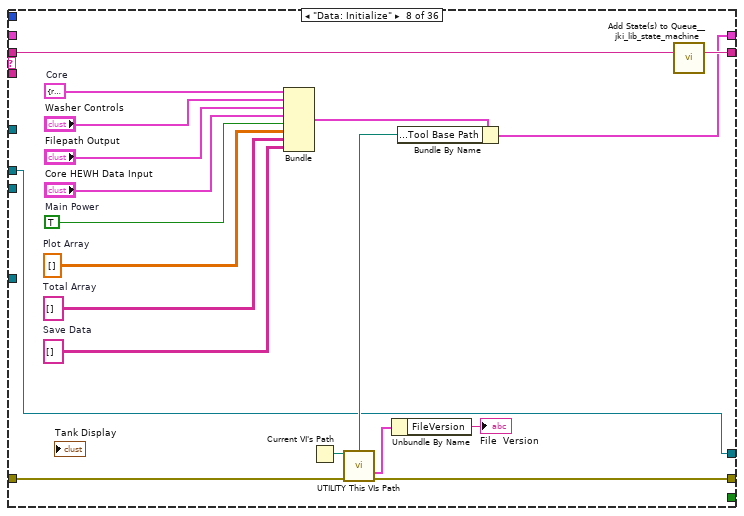
[diagram p17: hidden frame]
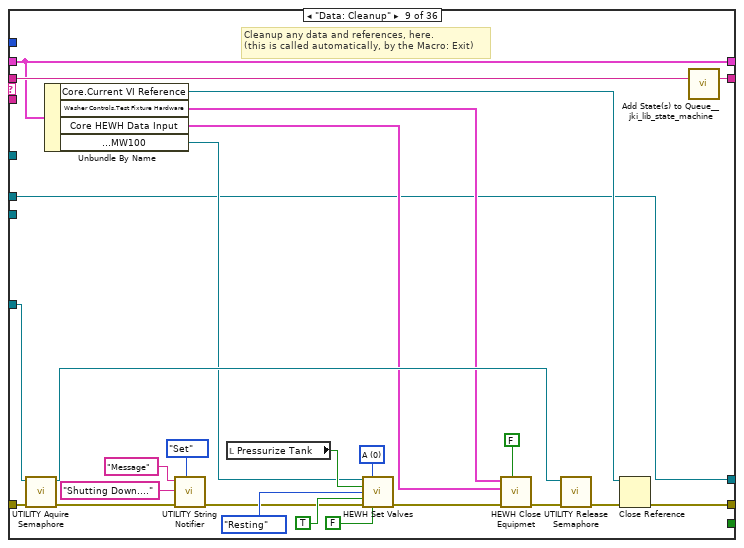
[diagram p18: hidden frame]
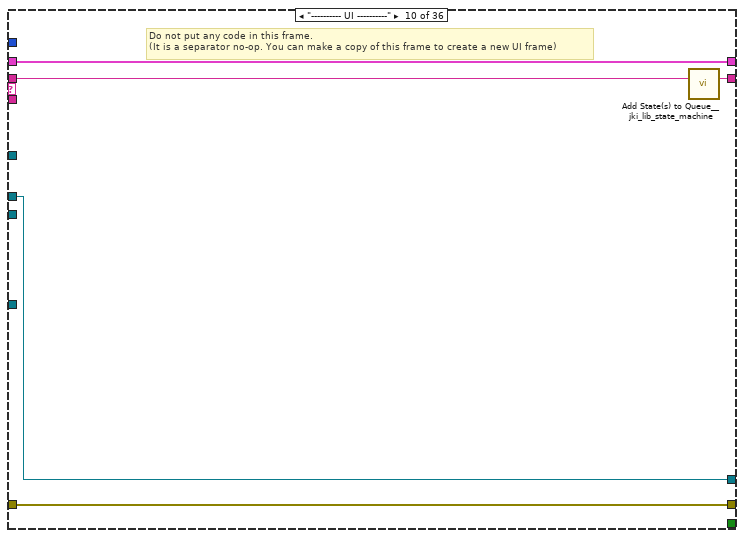
[diagram p19: hidden frame]
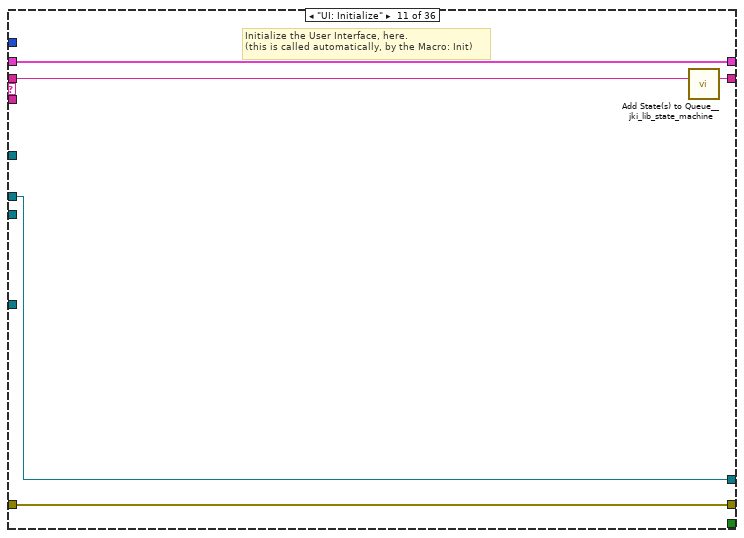
[diagram p20: hidden frame]
diagram:
  w18 = TRUE  # Update  Cycle Count
  n1 = flat-sequence {
    tunnel: "Error In" -> [w28]
    tunnel: [w28] -> w19
    frame #0 {
      w27 = FALSE ("Full Cutout")
      n2 = local write "Timer Reset"(w27) -> ()
      n3 = local write "Draw Complete"(w27) -> ()
      n4 = local write "Start Draw"(w27) -> ()
      n5 = local write "Start Test"(w27) -> ()
      n6 = local write "Shutdown"(w27) -> ()
    }
  }
  n7 = call <vilib>:"Obtain Semaphore Reference.vi"("error in (no error)"=w19, "name (unnamed)"="MW100") -> ("error out"=w17:errorcluster, "semaphore"=w21:T43)  [unwired: 3 in, 1 out]
  n8 = Create User Event(user event datatype=w18, error in=w17) -> (user event=w15:refnum<user-event>, error out=w7:errorcluster)
  n9 = register-events(w15) -> (reference out=w16:refnum<event-registration>)  [unwired: 2 in, 1 out]
  n10 = call "GEA2 Initialize.vi"("Board Index"=0, "Source Address"=u8 128, "error in"=w7) -> ("GEA2 Reference Out"=w11:refnum<k24>, "error out"=w10:errorcluster)  [unwired: 10 in, 1 out]
  n11 = call "GEA2 Register for Events.vi"("GEA2 Reference In"=w11, "Error In"=w10) -> ("GEA2 Reference Out"=w5:refnum<k24>, "GEA2 Event Registration"=w4:refnum<event-registration>, "Error Out"=w6:errorcluster)  [unwired: 11 in]
  n12 = call <vilib>:"Add State(s) to Queue__jki_lib_state_machine.vi"("State(s) in (\"\")"="Macro: Initialize") -> ("States Out"=w24:string)  [unwired: 14 in]
  n13 = while "Main RLT Event" {
    shift-right: [w42] -> _
    shift-left: _ -> [w41]
    shift-right: [w45] -> w3
    shift-left: w6 -> [w39]
    shift-right: [w44] -> _
    shift-left: w24 -> [w46]
    shift-right: [w35] -> _
    shift-left: string[] [] -> [w37]
    tunnel: w21 -> [w34]
    tunnel: w16 -> [w32]
    tunnel: w5 -> [w31]
    tunnel: w4 -> [w30]
    tunnel: [w29] -> w1
    i -> [w33]
    stop <- w43 stop-if-true
    w40 = 1000  # Timeout
    # "Main RLT Event"
    n14 = call <vilib>:"Parse State Queue__jki_lib_state_machine.vi"("State Queue"=w46, "Error In (no error)"=w39) -> ("Remaining States"=w48:string, "Current State"=w36:string, "Arguments"=w47:string)  [unwired: 11 in]
    n15 = case shown="\"Get Data\"" w36 {
      selector: w36 -> [_ _ w112 _ _ _ _ _ _ _ _ _ _ _ _ _ _ _ _ _ _ _ _ _ _ _ _ _ _ _ _ _ _ _ _ _]
      tunnel: w48 -> [w61 w110 w116 w135 w142 w150 w155 w174 w200 w205 w210 w217 w229 w256 w269 w279 w296 w310 w321 w344 w364 w384 w404 w416 w430 w435 w441 w452 w457 w467 w478 w505 w524 w542 w552 w577]
      tunnel: w47 -> [_ _ _ _ _ _ _ _ _ _ _ w212 w223 _ _ _ _ _ _ _ _ _ _ _ _ _ _ _ _ _ _ _ _ _ _ _]
      tunnel: w41 -> [w59 w107 w114 w126 w139 w148 w152 _ w198 w202 w208 w215 w225 w254 w262 w272 w283 w307 w313 w325 w348 w368 w388 w414 w418 w432 w438 w449 w454 w461 w476 w491 w518 w539 w549 w575]
      tunnel: [w58 w108 w118 w132 errorcluster {"status"=FALSE, "code"=0, "source"=""} ("error out") w147 w153 w157 w186 w203 w207 w213 w226 w253 w257 w275 w285 w304 w316 w328 w351 w371 w391 w409 w420 w433 w439 w450 w455 w464 w469 w493 w521 w540 w550 w568] -> w45
      tunnel: w39 -> [w57 w108 w117 w132 w138 w147 w153 w158 w184 w203 w207 w214 w227 w253 w258 w274 w289 w303 w319 w331 w354 w374 w394 w409 w421 w433 w439 w450 w455 w465 w470 w495 w512 w540 w550 w569]
      tunnel: [w60 w109 w115 w134 w141 w149 w154 w173 w199 w204 w209 w216 w228 w255 w268 w278 w295 w309 w320 w343 w363 w383 w403 w415 w429 w434 w440 w451 w456 w466 w477 w504 w523 w541 w551 w576] -> w44
      tunnel: [_ _ _ _ _ w144 _ _ _ _ _ _ _ _ _ _ _ _ _ _ _ _ _ _ _ _ _ _ _ _ _ _ _ _ _ _] -> w43
      tunnel: [w56 w107 w114 w133 w139 w148 w152 w160 w198 w202 w208 w215 w225 w254 w261 w271 w283 w307 w313 w325 w348 w368 w388 w414 w418 w432 w438 w449 w454 w460 w476 w490 w517 w538 w549 w574] -> w42
      tunnel: w40 -> [w55 _ _ _ _ _ _ _ _ _ _ _ _ _ _ _ _ _ _ _ _ _ _ _ _ _ _ _ _ _ _ _ _ _ _ _]
      tunnel: w34 -> [_ _ _ _ _ _ _ _ w179 _ _ _ _ _ _ _ w287 w300 w315 w327 w350 w370 w390 _ _ _ _ _ _ _ _ w494 _ _ _ _]
      tunnel: w32 -> [w54 _ _ _ _ _ _ _ _ _ _ _ _ _ _ _ _ _ _ _ _ _ _ _ _ _ _ _ _ _ _ _ _ _ _ _]
      tunnel: w31 -> [w53 w106 w111 w123 w136 w143 w151 w156 w175 w201 w206 w211 w222 w252 w263 w273 w280 w297 w311 w323 w345 w365 w385 w408 w417 w431 w436 w442 w453 w458 w468 w479 w508 w525 w546 w565]
      tunnel: w30 -> [_ _ _ _ _ _ _ _ _ _ _ _ _ _ _ _ _ _ _ _ _ _ _ _ _ _ _ _ _ _ _ _ w507 _ _ _]
      tunnel: [w53 w106 w111 w123 w136 w143 w151 w156 w175 w201 w206 w211 w222 w252 w263 w273 w280 w297 w311 w323 w345 w365 w385 w408 w417 w431 w436 w442 w453 w458 w468 w479 w506 w525 w546 w565] -> w29
      frame "", "Idle" {
        n16 = event shown="[4] \"X-Axis\": Value Change" {
          selector: w54 -> [_ _ _ _ _ _ _]
          dyn-events: _ -> [_ _ _ _ _ _ _]
          timeout: w55 -> [_ _ _ _ _ _ _]
          tunnel: w61 -> [w67 w75 w81 w84 w91 w95 w104]
          tunnel: [w66 w74 w82 w85 w92 w96 w105] -> w60
          tunnel: w59 -> [w64 w72 w78 w86 w90 w94 w102]
          tunnel: [w65 w73 w80 w87 w89 w93 w103] -> w58
          tunnel: w57 -> [w65 w73 w80 w87 w89 w93 w103]
          tunnel: [w64 w72 w77 w86 w90 w94 w101] -> w56
          event Timeout {
            (unwired) "Check Condition\nSave Data"
            n17 = event-data() -> ()  [unwired: 1 in, 1 out]
            n18 = case shown="False" "Start Test" {
              tunnel: ["Elapsed Time\nGet General Info\nGet Data\nCheck Newfi\nShow Data\nCheck Condition" "Elapsed Time\nGet General Info\nGet Data\nCheck Newfi\nShow Data\nCheck Condition\nSave Data"] -> w63
              frame False {
              }
              frame True {
              }
            }
            n19 = call <vilib>:"Add State(s) to Queue__jki_lib_state_machine.vi"("State(s) in Front (\"\")"=w63, "State(s) in (\"\")"=w67) -> ("States Out"=w66:string)  [unwired: 13 in]
          }
          event Panel Close? {
            n20 = event-data() -> ()  [unwired: 1 in, 1 out]
            n21 = event-data("Discard?"=TRUE) -> ()  [unwired: 1 in, 1 out]
            n22 = call <vilib>:"Add State(s) to Queue__jki_lib_state_machine.vi"("State(s) in Front (\"\")"="Macro: Exit", "State(s) in (\"\")"=w75) -> ("States Out"=w74:string)  [unwired: 13 in]
          }
          event "HEWH Power": Value Change {
            n23 = event-data() -> ("NewVal"=w76:bool)  [unwired: 1 in, 5 out]
            n24 = Bundle By Name(cluster=w78, "Main Power"=w76) -> (w77:T50)
            n25 = call <vilib>:"Add State(s) to Queue__jki_lib_state_machine.vi"("State(s) in Front (\"\")"="Main Power" ("State(s) in Front (\"\")"), "State(s) in (\"\")"=w81) -> ("States Out"=w82:string)  [unwired: 13 in]
          }
          event "Reset Gallons": Value Change {
            n26 = event-data() -> ()  [unwired: 1 in, 6 out]
            n27 = call <vilib>:"Add State(s) to Queue__jki_lib_state_machine.vi"("State(s) in Front (\"\")"="Reset Totalizer" ("State(s) in Front (\"\")"), "State(s) in (\"\")"=w84) -> ("States Out"=w85:string)  [unwired: 13 in]
          }
          event "X-Axis": Value Change {
            n28 = event-data() -> ()  [unwired: 1 in, 6 out]
            n29 = call <vilib>:"Add State(s) to Queue__jki_lib_state_machine.vi"("State(s) in Front (\"\")"="Populate XY Axis", "State(s) in (\"\")"=w91) -> ("States Out"=w92:string)  [unwired: 13 in]
          }
          event "Y-Axis-1", "Y-Axis-2": Value Change {
            n30 = event-data() -> ()  [unwired: 1 in, 6 out]
            n31 = call <vilib>:"Add State(s) to Queue__jki_lib_state_machine.vi"("State(s) in Front (\"\")"="Populate XY Axis", "State(s) in (\"\")"=w95) -> ("States Out"=w96:string)  [unwired: 13 in]
          }
          event User Event {
            n32 = event-data() -> ()  [unwired: 1 in, 5 out]
            n33 = local read "Core HEWH Data out"() -> (w100:T29)
            n34 = Unbundle By Name(w100) -> ("Draw Count"=w99:i32, "Calc and Calibration"=w98:T40)
            n35 = Bundle By Name(cluster=w102, "Core HEWH Data Input.Draw Count"=w99, "Core HEWH Data Input.Calc and Calibration"=w98) -> (w101:T50)
            n36 = call <vilib>:"Add State(s) to Queue__jki_lib_state_machine.vi"("State(s) in (\"\")"=w104) -> ("States Out"=w105:string)  [unwired: 14 in]
          }
        }
      }
      frame "---------- Core ----------" {
        # "Do not put any code in this frame.\n(it is a separator no-op)"
        n37 = call <vilib>:"Add State(s) to Queue__jki_lib_state_machine.vi"("State(s) in (\"\")"=w110) -> ("States Out"=w109:string)  [unwired: 14 in]
      }
      frame Default {
        w121 = 42 items=["No error", "Argument error", "Memory is full", "Out of zone", "End of file", "File already open", "Generic file I/O error", "File not found", "File permission error", "Disk is full", "Duplicate path", "Too many files open", "System feature not enabled", "Resource file not found", "Cannot add resource", "Resource not found", "Image not found", "Image memory error", "Pen does not exist", "Config type invalid", "Config token not found", "Config parse error", "Config memory error", "Bad external code format", "Bad external code offset", "External code not present", "Null window", "Destroy window error", "Null menu", "Print aborted", "Bad print record", "Print driver error", "Windows error during printing", "Memory error during printing", "Print dialog error", "Generic print error", "Invalid device refnum", "Device not found", "Device parameter error", "Device unit error", "Cannot open device", "Device call aborted", "Generic error", "Cancelled by user", "Object ID too low", "Object ID too high", "Object not in heap", "Unknown heap", "Unknown object (invalid DefProc)", "Unknown object (DefProc not in table)", "Message out of range", "Invalid (null) method", "Unknown message", "Manager call not supported", "Bad address", "Network operation in progress", "Network operation timed out", "Connection is busy", "Network attribute not supported", "Network error", "Address in use", "System out of memory", "Connection aborted", "Connection refused", "Not connected", "Already connected", "Connection closed", "Initialization error (interapplication manager)", "Bad occurrence", "Wait on unbound occurrence handler", "Occurrence queue overflow", "Datalog type conflict", "Unused", "Unrecognized type (interapplication manager)", "Memory corrupt", "Failed to make temporary DLL", "Old CIN version", "Drag socket not found", "Failed to load drop-object", "Failed to register OLE object", "Failed to release OLE object", "Format specifier type mismatch", "Unknown format specifier", "Too few format specifiers", "Too many format specifiers", "Scan failed", "Newer CIN version", "Error converting to variant", "Runtime menu error", "Password tampered", "Variant attribute not found", "Incompatible variant data type", "Event data is not available", "Event Store is not present", "Occurrence is not found", "Event Queue is not created", "Event info is not available", "Refnum passed is NULL", "Error retrieving Class GUID", "Error retrieving CoClass GUID", "Error retrieving TypeLib GUID.", "Bad built application magic bytes.", "Specific driver is different from the specific driver associated with the Logical Name.", "There is no session opened to the class driver.", "Max Error", "MAX - Error with config objects", "MAX - Error loading configuration", "MAX - Group not supported"]
        # "Current State"
        # "Do not delete, rename, or modify this frame.\n(this is used to capture unhandled states and typos)"
        # "Handle mistyped state name (developer tool)"
        n38 = Format Into String(format string="Software Exception: Unhandled State \"%s\"." ("message"), error in=w117, w112) -> (resulting string=w120:string, error out=w119:errorcluster)  [unwired: 1 in]
        n39 = call <vilib>:"Error Cluster From Error Code.vi"("show call chain? (False)"=TRUE, "error in (no error)"=w119, "error message (\"\")"=w120, "error code (0)"=w121) -> ("error out"=w118:errorcluster)  [unwired: 5 in]
        n40 = call <vilib>:"Add State(s) to Queue__jki_lib_state_machine.vi"("State(s) in (\"\")"=w116) -> ("States Out"=w115:string)  [unwired: 14 in]
      }
      frame "Initialize Core Data" {
        # "Do not delete, rename, or modify this frame.\n(this is used to determine panel behavior on exit)"
        # "originally closed?"
        # "exe?"
        # "If panel starts closed or is an EXE, then close it when we exit"
        n41 = property class="VI"() -> ("Front Panel.Open"=w131:bool)  [unwired: 2 in, 2 out]
        n42 = property class="App"() -> ("App.Kind"=w130:T44)  [unwired: 2 in, 2 out]
        n43 = control-ref of="Current VI Reference"() -> (w124:refnum<vi>)
        n44 = Not(x=w131) -> (.not. x?=w128:bool)
        n45 = Equal?(x=w130, y=T44."Run Time System" ("Application:Kind")) -> (x = y?=w127:bool)
        n46 = Or(x=w128, y=w127) -> (x .or. y?=w125:bool)
        n47 = Bundle By Name(cluster=w126, "Core.Current VI Reference"=w124, "Core.Close Panel on Exit?"=w125) -> (w133:T50)
        n48 = call <vilib>:"Add State(s) to Queue__jki_lib_state_machine.vi"("State(s) in (\"\")"=w135) -> ("States Out"=w134:string)  [unwired: 14 in]
      }
      frame "Error Handler" {
        # "Unhandled Error -- Display it"
        # "Handle any errors here.\nYou can also output any states to clean-up after errors occur"
        # "Clear error"
        n49 = call <vilib>:"General Error Handler.vi"("error in (no error)"=w138) -> ()  [unwired: 10 in, 5 out]
        n50 = call <vilib>:"Add State(s) to Queue__jki_lib_state_machine.vi"("State(s) in Front (\"\")"="/* Post Error States", "State(s) in (\"\")"=w142) -> ("States Out"=w141:string)  [unwired: 13 in]
      }
      frame "Exit" {
        w144 = TRUE
        n51 = call "UTILITY Boolean Notifier.vi"("Status"=UTILITY_Notifier."Set", "Set Status"=w144, "name (unnamed)"="Stop Custom Draw") -> ()  [unwired: 7 in, 2 out]
        n52 = call <vilib>:"Add State(s) to Queue__jki_lib_state_machine.vi"("State(s) in (\"\")"=w150) -> ("States Out"=w149:string)  [unwired: 14 in]
        "Shutdown" <- w144
      }
      frame "---------- Data ----------" {
        # "Do not put any code in this frame.\n(It is a separator no-op. You can make a copy of this frame to create a new Data frame)"
        n53 = call <vilib>:"Add State(s) to Queue__jki_lib_state_machine.vi"("State(s) in (\"\")"=w155) -> ("States Out"=w154:string)  [unwired: 14 in]
      }
      frame "Data: Initialize" {
        w166 = string[][] []  # Total Array
        w165 = string[][] []  # Save Data
        w167 = dbl[][] []  # Plot Array
        w172 = T51 {"Current VI Reference"=refnum, "Close Panel on Exit?"=FALSE}  # Core
        w169 = TRUE  # Main Power
        n54 = Bundle("Core"=w172, "Washer Controls"="Washer Controls", "Filepath Output"="Filepath Output", "Core HEWH Data Input"="Core HEWH Data Input", "Main Power"=w169, "Plot Array"=w167, "Total Array"=w166, "Save Data"=w165) -> (w161:T50)  [unwired: 1 in]
        n55 = Current VI's Path() -> (path=w162:path)
        n56 = call "UTILITY This VIs Path.vi"("path"=w162, "error in (no error)"=w158) -> ("Folder Path"=w159:path, "FileVersionInfo Out"=w163:T14, "error out"=w157:errorcluster)  [unwired: 7 in, 4 out]
        n57 = Unbundle By Name(w163) -> ("FileVersion"=→"File  Version":string)
        n58 = Bundle By Name(cluster=w161, "Filepath Output.General Setup Paths.Tool Base Path"=w159) -> (w160:T50)
        n59 = call <vilib>:"Add State(s) to Queue__jki_lib_state_machine.vi"("State(s) in (\"\")"=w174) -> ("States Out"=w173:string)  [unwired: 14 in]
      }
      frame "Data: Cleanup" {
        w195 = u16 0 items=["A", "B", "C", "D"] ("Valve Bank")
        # "Cleanup any data and references, here.\n(this is called automatically, by the Macro: Exit)"
        n60 = call "UTILITY Aquire Semaphore.vi"("error in (no error)"=w184, "Refnum in"=w179) -> ("error out"=w183:errorcluster, "Refnum out"=w180:T43)  [unwired: 7 in, 1 out]
        n61 = Unbundle By Name(w198) -> ("Core.Current VI Reference"=w185:refnum<vi>, "Washer Controls.Test Fixture Hardware"=w178:T4, "Core HEWH Data Input"=w176:T29, "Washer Controls.Test Fixture Hardware.Analog Data.Yokogawa.MW100"=w177:refnum<visa-resource-name>)
        n62 = call "UTILITY String Notifier.vi"("Status"=UTILITY_Notifier."Set", "error in (no error)"=w183, "Set Status"="Shutting Down....", "name (unnamed)"="Message") -> ("error out"=w187:errorcluster)  [unwired: 6 in, 1 out]
        n63 = local read "Pressurize Tank"() -> (w191:bool)
        n64 = call "HEWH Set Valves.vi"("VISA session"=w177, "Station ID"=w195, "Pressurize Tank?"=w191, "Valve Bank Setting"=HEWH_Valve_Bank_Positions."Resting", "Stop Intellifaucet?"=TRUE, "Error In"=w187, "Start Intellifaucet?"=FALSE) -> ("Error Out"=w193:errorcluster)  [unwired: 7 in, 1 out]
        n65 = call "HEWH Close Equipmet.vi"("Use Agilent?"=FALSE, "Error In"=w193, "Core HEWH Data"=w176, "Test Fixture Hardware In"=w178) -> ("Error Out"=w182:errorcluster)  [unwired: 6 in, 1 out]
        n66 = call "UTILITY Release Semaphore.vi"("error in (no error)"=w182, "Refnum in"=w180) -> ("error out"=w181:errorcluster)  [unwired: 9 in]
        n67 = Close Reference(reference=w185, error in (no error)=w181) -> (error out=w186:errorcluster)
        n68 = call <vilib>:"Add State(s) to Queue__jki_lib_state_machine.vi"("State(s) in (\"\")"=w200) -> ("States Out"=w199:string)  [unwired: 14 in]
      }
      frame "---------- UI ----------" {
        # "Do not put any code in this frame.\n(It is a separator no-op. You can make a copy of this frame to create a new UI frame)"
        n69 = call <vilib>:"Add State(s) to Queue__jki_lib_state_machine.vi"("State(s) in (\"\")"=w205) -> ("States Out"=w204:string)  [unwired: 14 in]
      }
      frame "UI: Initialize" {
        # "Initialize the User Interface, here.\n(this is called automatically, by the Macro: Init)"
        n70 = call <vilib>:"Add State(s) to Queue__jki_lib_state_machine.vi"("State(s) in (\"\")"=w210) -> ("States Out"=w209:string)  [unwired: 14 in]
      }
      frame "UI: Cursor Set" {
        # "Argument"
        # "Set and Unset Cursor Busy.\n(Usage: \"UI: Cursor Set >> Busy|Idle\")"
        n71 = case shown="\"Idle\", Default" w212 {
          tunnel: w214 -> [w219 w221]
          tunnel: [w218 w220] -> w213
          frame "Idle", Default {
            n72 = call <vilib>:"Unset Busy.vi"("error in (no error)"=w219) -> ("error out"=w218:errorcluster)  [unwired: 10 in]
          }
          frame "Busy" {
            n73 = call <vilib>:"Set Busy.vi"("error in (no error)"=w221) -> ("error out"=w220:errorcluster)  [unwired: 9 in, 1 out]
          }
        }
        n74 = call <vilib>:"Add State(s) to Queue__jki_lib_state_machine.vi"("State(s) in (\"\")"=w217) -> ("States Out"=w216:string)  [unwired: 14 in]
      }
      frame "UI: Front Panel State" {
        # "Argument"
        # "Set Front Panel Open or Closed\n(Usage: \"UI: Front Panel State >> Open|Close\")"
        n75 = Unbundle By Name(w225) -> ("Core.Current VI Reference"=w224:refnum<vi>)
        n76 = case shown="\"Open\", Default" w223 {
          tunnel: w227 -> [w233 w246]
          tunnel: [w235 w247] -> w226
          tunnel: w224 -> [w234 w244]
          frame "Open", Default {
            n77 = property class="VI"(reference=w234, error in=w233) -> (reference out=w231:refnum<vi>, error out=w232:errorcluster, "Front Panel.Open"=w230:bool)
            n78 = case shown="False" w230 {
              tunnel: [w238 w241] -> w235
              tunnel: w232 -> [w237 w241]
              tunnel: w231 -> [w236 _]
              frame False {
                n79 = invoke class="VI" method="FP.Open"(reference=w236, error in=w237, "Activate"=TRUE, "State"=T47."Standard") -> (error out=w238:errorcluster)  [unwired: 1 in, 4 out]
              }
              frame True {
              }
            }
          }
          frame "Close" {
            n80 = property class="VI"(reference=w244, error in=w246) -> (reference out=w243:refnum<vi>, error out=w245:errorcluster, "Front Panel.Open"=w242:bool)
            n81 = case shown="True" w242 {
              tunnel: [w248 w251] -> w247
              tunnel: w245 -> [w248 w250]
              tunnel: w243 -> [_ w249]
              frame False {
              }
              frame True {
                n82 = invoke class="VI" method="FP.Close"(reference=w249, error in=w250) -> (error out=w251:errorcluster)  [unwired: 1 in, 2 out]
              }
            }
          }
        }
        n83 = call <vilib>:"Add State(s) to Queue__jki_lib_state_machine.vi"("State(s) in (\"\")"=w229) -> ("States Out"=w228:string)  [unwired: 14 in]
      }
      frame "Read Configuration File" {
        n84 = call "UTILITY Initialize Front Panel Controls.vi"() -> ()  [unwired: 10 in, 2 out]
        n85 = call <vilib>:"Add State(s) to Queue__jki_lib_state_machine.vi"("State(s) in (\"\")"=w256) -> ("States Out"=w255:string)  [unwired: 14 in]
      }
      frame "File Setup" {
        n86 = Unbundle By Name(w262) -> ("Filepath Output"=w266:T1, "Core HEWH Data Input.LV Program"=w264:T41, "Washer Controls"=w265:T3)
        n87 = call "Save File DOE File Setup.vi"("Filepath In"=w266, 1:w264, "Washer Controls In"=w265, "error in (no error)"=w258, "Config State"=Save_File_DOE_Configuration_State."Open Front Panel") -> ("Washer Controls Out"=w259:T3, "Filepath Out"=w260:T1, "error out"=w257:errorcluster)  [unwired: 12 in]
        n88 = Bundle By Name(cluster=w262, "Washer Controls"=w259, "Filepath Output"=w260) -> (w261:T50)
        n89 = call <vilib>:"Add State(s) to Queue__jki_lib_state_machine.vi"("State(s) in (\"\")"=w269) -> ("States Out"=w268:string)  [unwired: 14 in]
      }
      frame "Test Setup" {
        n90 = Unbundle By Name(w272) -> ("Core HEWH Data Input"=w276:T29)
        n91 = call "HEWH Dispense Schedule.vi"("Core HEWH Data Input"=w276, "Hide PreDraw Tab"=FALSE, "error in (no error)"=w274) -> ("Core HEWH Data Input Out"=w270:T29, "error out"=w275:errorcluster)  [unwired: 11 in]
        n92 = Bundle By Name(cluster=w272, "Core HEWH Data Input"=w270) -> (w271:T50)
        n93 = call <vilib>:"Add State(s) to Queue__jki_lib_state_machine.vi"("State(s) in (\"\")"=w279) -> ("States Out"=w278:string)  [unwired: 14 in]
      }
      frame "Initialize Equipment" {
        n94 = Unbundle By Name(w283) -> ("Washer Controls.Test Fixture Hardware"=w282:T4, "Core HEWH Data Input"=w281:T29)
        n95 = call "UTILITY Aquire Semaphore.vi"("error in (no error)"=w289, "Refnum in"=w287) -> ("error out"=w288:errorcluster, "Refnum out"=w284:T43)  [unwired: 7 in, 1 out]
        n96 = call "HEWH Initialize Equipmet.vi"("Use Agilent?"=FALSE, "Error In"=w288, "Core HEWH Data"=w281, "Test Fixture Hardware"=w282) -> ("Error Out"=w290:errorcluster)  [unwired: 6 in, 1 out]
        n97 = call "UTILITY String Notifier.vi"("Status"=UTILITY_Notifier."Set", "error in (no error)"=w290, "Set Status"="", "name (unnamed)"="Message") -> ("error out"=w286:errorcluster)  [unwired: 6 in, 1 out]
        n98 = call "UTILITY Release Semaphore.vi"("error in (no error)"=w286, "Refnum in"=w284) -> ("error out"=w285:errorcluster)  [unwired: 9 in]
        n99 = call <vilib>:"Add State(s) to Queue__jki_lib_state_machine.vi"("State(s) in (\"\")"=w296) -> ("States Out"=w295:string)  [unwired: 14 in]
      }
      frame "Main Power" {
        n100 = Unbundle By Name(w307) -> ("Washer Controls.Test Fixture Hardware.Analog Data.Yokogawa.MW100"=w299:refnum<visa-resource-name>, "Main Power"=w306:bool)
        n101 = call "UTILITY Aquire Semaphore.vi"("error in (no error)"=w303, "Refnum in"=w300) -> ("error out"=w302:errorcluster, "Refnum out"=w301:T43)  [unwired: 7 in, 1 out]
        n102 = Boolean To (0,1)(Boolean=w306) -> (0, 1=w308:i16)
        n103 = call "INTELLIFAUCET DO Control.vi"("VISA session"=w299, "HEWH MW100 Channel Numbers"=T49 "047", "Relay Status (0:CLOSED)"=w308, "Error In"=w302) -> ("error out"=w305:errorcluster)  [unwired: 9 in, 2 out]
        n104 = call "UTILITY Release Semaphore.vi"("error in (no error)"=w305, "Refnum in"=w301) -> ("error out"=w304:errorcluster)  [unwired: 9 in]
        n105 = call <vilib>:"Add State(s) to Queue__jki_lib_state_machine.vi"("State(s) in (\"\")"=w310) -> ("States Out"=w309:string)  [unwired: 14 in]
      }
      frame "Reset Totalizer" {
        n106 = Unbundle By Name(w313) -> ("Washer Controls.Test Fixture Hardware.Analog Data.Yokogawa.MW100"=w312:refnum<visa-resource-name>)
        n107 = call "UTILITY Aquire Semaphore.vi"("error in (no error)"=w319, "Refnum in"=w315) -> ("error out"=w318:errorcluster, "Refnum out"=w314:T43)  [unwired: 7 in, 1 out]
        n108 = call "HEWH Reset MW100.vi"("error in (no error)"=w318, "MW100 VISA In"=w312) -> ("error out"=w317:errorcluster)  [unwired: 8 in, 1 out]
        n109 = call "UTILITY Release Semaphore.vi"("error in (no error)"=w317, "Refnum in"=w314) -> ("error out"=w316:errorcluster)  [unwired: 9 in]
        n110 = call <vilib>:"Add State(s) to Queue__jki_lib_state_machine.vi"("State(s) in (\"\")"=w321) -> ("States Out"=w320:string)  [unwired: 14 in]
      }
      frame "Set Valve Bank 1" {
        w340 = u16 0 items=["A", "B", "C", "D"] ("Valve Bank")
        n111 = call "UTILITY Aquire Semaphore.vi"("error in (no error)"=w331, "Refnum in"=w327) -> ("error out"=w330:errorcluster, "Refnum out"=w326:T43)  [unwired: 7 in, 1 out]
        n112 = Unbundle By Name(w325) -> ("Washer Controls.Test Fixture Hardware.Analog Data.Yokogawa.MW100"=w324:refnum<visa-resource-name>)
        n113 = call "UTILITY String Notifier.vi"("Status"=UTILITY_Notifier."Set", "error in (no error)"=w330, "Set Status"="Initializing Valve Bank A....", "name (unnamed)"="Message") -> ("error out"=w333:errorcluster)  [unwired: 6 in, 1 out]
        n114 = call "YKMW100 VF0 Relay Status.vi"("VISA session"=w324, "Error In"=w333) -> ("dup VISA session"=w342:refnum<visa-resource-name>, "Control Relay ON (Supplying Power to Unit)"=w322:bool, "error out"=w341:errorcluster)  [unwired: 9 in, 2 out]
        n115 = local write "HEWH Power"(w322) -> ()
        n116 = local read "Pressurize Tank"() -> (w336:bool)
        n117 = call "HEWH Set Valves.vi"("VISA session"=w342, "Station ID"=w340, "Pressurize Tank?"=w336, "Valve Bank Setting"=HEWH_Valve_Bank_Positions."Heating", "Stop Intellifaucet?"=TRUE, "Error In"=w341, "Start Intellifaucet?"=FALSE) -> ("Error Out"=w329:errorcluster)  [unwired: 7 in, 1 out]
        n118 = call "UTILITY Release Semaphore.vi"("error in (no error)"=w329, "Refnum in"=w326) -> ("error out"=w328:errorcluster)  [unwired: 9 in]
        n119 = call <vilib>:"Add State(s) to Queue__jki_lib_state_machine.vi"("State(s) in (\"\")"=w344) -> ("States Out"=w343:string)  [unwired: 14 in]
      }
      frame "Set Valve Bank 2" {
        w362 = u16 1 items=["A", "B", "C", "D"] ("Valve Bank")
        n120 = call "UTILITY Aquire Semaphore.vi"("error in (no error)"=w354, "Refnum in"=w350) -> ("error out"=w353:errorcluster, "Refnum out"=w349:T43)  [unwired: 7 in, 1 out]
        n121 = call "UTILITY String Notifier.vi"("Status"=UTILITY_Notifier."Set", "error in (no error)"=w353, "Set Status"="Initializing Valve Bank B....", "name (unnamed)"="Message") -> ("error out"=w346:errorcluster)  [unwired: 6 in, 1 out]
        n122 = Unbundle By Name(w348) -> ("Washer Controls.Test Fixture Hardware.Analog Data.Yokogawa.MW100"=w347:refnum<visa-resource-name>)
        n123 = local read "Pressurize Tank"() -> (w358:bool)
        n124 = call "HEWH Set Valves.vi"("VISA session"=w347, "Station ID"=w362, "Pressurize Tank?"=w358, "Valve Bank Setting"=HEWH_Valve_Bank_Positions."Heating", "Stop Intellifaucet?"=TRUE, "Error In"=w346, "Start Intellifaucet?"=FALSE) -> ("Error Out"=w352:errorcluster)  [unwired: 7 in, 1 out]
        n125 = call "UTILITY Release Semaphore.vi"("error in (no error)"=w352, "Refnum in"=w349) -> ("error out"=w351:errorcluster)  [unwired: 9 in]
        n126 = call <vilib>:"Add State(s) to Queue__jki_lib_state_machine.vi"("State(s) in (\"\")"=w364) -> ("States Out"=w363:string)  [unwired: 14 in]
      }
      frame "Set Valve Bank 3" {
        w382 = u16 2 items=["A", "B", "C", "D"] ("Valve Bank")
        n127 = call "UTILITY Aquire Semaphore.vi"("error in (no error)"=w374, "Refnum in"=w370) -> ("error out"=w373:errorcluster, "Refnum out"=w369:T43)  [unwired: 7 in, 1 out]
        n128 = call "UTILITY String Notifier.vi"("Status"=UTILITY_Notifier."Set", "error in (no error)"=w373, "Set Status"="Initializing Valve Bank C....", "name (unnamed)"="Message") -> ("error out"=w366:errorcluster)  [unwired: 6 in, 1 out]
        n129 = Unbundle By Name(w368) -> ("Washer Controls.Test Fixture Hardware.Analog Data.Yokogawa.MW100"=w367:refnum<visa-resource-name>)
        n130 = local read "Pressurize Tank"() -> (w378:bool)
        n131 = call "HEWH Set Valves.vi"("VISA session"=w367, "Station ID"=w382, "Pressurize Tank?"=w378, "Valve Bank Setting"=HEWH_Valve_Bank_Positions."Heating", "Stop Intellifaucet?"=TRUE, "Error In"=w366, "Start Intellifaucet?"=FALSE) -> ("Error Out"=w372:errorcluster)  [unwired: 7 in, 1 out]
        n132 = call "UTILITY Release Semaphore.vi"("error in (no error)"=w372, "Refnum in"=w369) -> ("error out"=w371:errorcluster)  [unwired: 9 in]
        n133 = call <vilib>:"Add State(s) to Queue__jki_lib_state_machine.vi"("State(s) in (\"\")"=w384) -> ("States Out"=w383:string)  [unwired: 14 in]
      }
      frame "Set Valve Bank 4" {
        w402 = u16 3 items=["A", "B", "C", "D"] ("Valve Bank")
        n134 = call "UTILITY Aquire Semaphore.vi"("error in (no error)"=w394, "Refnum in"=w390) -> ("error out"=w393:errorcluster, "Refnum out"=w389:T43)  [unwired: 7 in, 1 out]
        n135 = call "UTILITY String Notifier.vi"("Status"=UTILITY_Notifier."Set", "error in (no error)"=w393, "Set Status"="Initializing Valve Bank D....", "name (unnamed)"="Message") -> ("error out"=w386:errorcluster)  [unwired: 6 in, 1 out]
        n136 = Unbundle By Name(w388) -> ("Washer Controls.Test Fixture Hardware.Analog Data.Yokogawa.MW100"=w387:refnum<visa-resource-name>)
        n137 = local read "Pressurize Tank"() -> (w398:bool)
        n138 = call "HEWH Set Valves.vi"("VISA session"=w387, "Station ID"=w402, "Pressurize Tank?"=w398, "Valve Bank Setting"=HEWH_Valve_Bank_Positions."Heating", "Stop Intellifaucet?"=TRUE, "Error In"=w386, "Start Intellifaucet?"=FALSE) -> ("Error Out"=w392:errorcluster)  [unwired: 7 in, 1 out]
        n139 = call "UTILITY Release Semaphore.vi"("error in (no error)"=w392, "Refnum in"=w389) -> ("error out"=w391:errorcluster)  [unwired: 9 in]
        n140 = call <vilib>:"Add State(s) to Queue__jki_lib_state_machine.vi"("State(s) in (\"\")"=w404) -> ("States Out"=w403:string)  [unwired: 14 in]
      }
      frame "Populate XY Axis" {
        n141 = Unbundle By Name(w414) -> ("Save Data"=w413:string[][])
        n142 = Index Array(array=w413, index (row)=0 ("disabled index (col)")) -> (element=w412:string[])  [unwired: 1 in]
        n143 = Index Array(array=w413, index (row)=0 ("disabled index (col)")) -> (element=w411:string[])  [unwired: 1 in]
        n144 = Index Array(array=w413, index (row)=0 ("disabled index (col)")) -> (element=w410:string[])  [unwired: 1 in]
        n145 = property on="X-Axis" class="CmbBox"("Strings[]"=w412) -> ()  [unwired: 2 in, 2 out]
        n146 = property on="Y-Axis-1" class="CmbBox"("Strings[]"=w411) -> ()  [unwired: 2 in, 2 out]
        n147 = property on="Y-Axis-2" class="CmbBox"("Strings[]"=w410) -> ()  [unwired: 2 in, 2 out]
        n148 = call <vilib>:"Add State(s) to Queue__jki_lib_state_machine.vi"("State(s) in (\"\")"=w416) -> ("States Out"=w415:string)  [unwired: 14 in]
      }
      frame "Start Loops" {
        n149 = Unbundle By Name(w418) -> ("Washer Controls.Test Fixture Hardware.Analog Data.Yokogawa.MW100"=→"MW100":refnum<visa-resource-name>)
        n150 = call "UTILITY Boolean Notifier.vi"("Status"=UTILITY_Notifier."Set", "error in (no error)"=w421, "Set Status"="Start UI Loop", "name (unnamed)"="Start UI Loop") -> ("error out"=w423:errorcluster)  [unwired: 6 in, 1 out]
        n151 = call "UTILITY Boolean Notifier.vi"("Status"=UTILITY_Notifier."Set", "error in (no error)"=w423, "Set Status"="Pressurize Tank", "name (unnamed)"="Pressurize Tank?") -> ("error out"=w420:errorcluster)  [unwired: 6 in, 1 out]
        n152 = call <vilib>:"Add State(s) to Queue__jki_lib_state_machine.vi"("State(s) in (\"\")"=w430) -> ("States Out"=w429:string)  [unwired: 14 in]
      }
      frame "---------- Macro ----------" {
        # "Do not put any code in this frame.\n(It is a separator no-op. You can make a copy of this frame to create a new Macro frame)"
        n153 = call <vilib>:"Add State(s) to Queue__jki_lib_state_machine.vi"("State(s) in (\"\")"=w435) -> ("States Out"=w434:string)  [unwired: 14 in]
      }
      frame "Macro: Initialize" {
        (unwired) "Data: Initialize\nInitialize Core Data\nUI: Initialize\nUI: Front Panel State >> Open\n\nInitialize Equipment\nMain Power\nReset Totalizer\nSet Valve Bank 1\nPopulate XY Axis\nStart Loops"  # Data: Initialize Initialize Core Data UI: Initialize UI: Front Panel State >> Open  Initialize Equipment Main Power Reset Totalizer Set Valve Bank 1 Populate XY Axis Start Loops
        w437 = "Data: Initialize\nInitialize Core Data\nUI: Initialize\nUI: Front Panel State >> Open\nFile Setup\nTest Setup\nInitialize Equipment\nMain Power\nReset Totalizer\nSet Valve Bank 1\nStart Loops\nElapsed Time\nGet General Info\nGet Data\nCheck Newfi\nShow Data\nCheck Condition\nPopulate XY Axis"  # Data: Initialize Initialize Core Data UI: Initialize UI: Front Panel State >> Open File Setup Test Setup Initialize Equipment Main Power Reset Totalizer Set Valve Bank 1 Start Loops Elapsed Time Get General Info Get Data Check Newfi Show Data Check Condition Populate XY Axis
        n154 = call <vilib>:"Add State(s) to Queue__jki_lib_state_machine.vi"("State(s) in Front (\"\")"=w437, "State(s) in (\"\")"=w441) -> ("States Out"=w440:string)  [unwired: 13 in]
      }
      frame "Macro: Exit" {
        # "Exit Macro\n(This is called once, when the VI exits)"
        n155 = Unbundle By Name(w449) -> ("Core.Close Panel on Exit?"=w448:bool)
        n156 = Select(t="UI: Front Panel State >> Close", s=w448, f="") -> (s? t:f=w445:string)
        n157 = call <vilib>:"Add State(s) to Queue__jki_lib_state_machine.vi"("State(s) in (\"\")"=w445, "State(s) at Back (\"\")"="Data: Cleanup\nExit") -> ("States Out"=w443:string)  [unwired: 13 in]
        n158 = call <vilib>:"Add State(s) to Queue__jki_lib_state_machine.vi"("State(s) in Front (\"\")"=w443, "State(s) in (\"\")"=w452) -> ("States Out"=w451:string)  [unwired: 13 in]
      }
      frame "---------- New Category ----------" {
        # "Template Separator\n(You can make a copy of, or modify, this frame)"
        n159 = call <vilib>:"Add State(s) to Queue__jki_lib_state_machine.vi"("State(s) in (\"\")"=w457) -> ("States Out"=w456:string)  [unwired: 14 in]
      }
      frame "Elapsed Time" {
        n160 = call "UTILITY Elapsed Time.vi"("error in (no error)"=w465) -> ("error out"=w464:errorcluster, "Main Loop Rate"=→"Main Loop Rate":dbl, "Elapsed Time"=→"Elapsed Time":dbl, "Total Array"=w459:string[][])  [unwired: 6 in, 1 out]
        n161 = Bundle By Name(cluster=w461, "Total Array"=w459) -> (w460:T50)
        n162 = call <vilib>:"Add State(s) to Queue__jki_lib_state_machine.vi"("State(s) in (\"\")"=w467) -> ("States Out"=w466:string)  [unwired: 14 in]
      }
      frame "Get General Info" {
        n163 = call "HEWH GET General Information.vi"("Stop Custom Draw"="Stop Custom Draw", "error in (no error)"=w470) -> ("UI Loop Status"=→"UI Loop Status":bool, "Stop Draw Status"=→"Stop Draw Status":bool, "Pressurize Tank Status"=→"Pressurize Tank Status":bool, "Message"=→"Message":string, "error out"=w469:errorcluster)  [unwired: 13 in]
        n164 = call <vilib>:"Add State(s) to Queue__jki_lib_state_machine.vi"("State(s) in (\"\")"=w478) -> ("States Out"=w477:string)  [unwired: 14 in]
      }
      frame "Get Data" {
        n165 = Unbundle By Name(w491) -> ("Total Array"=w489:string[][], "Washer Controls.Test Fixture Hardware"=w482:T4, "Core HEWH Data Input"=w492:T29)
        n166 = call "UTILITY Aquire Semaphore.vi"("error in (no error)"=w495, "Refnum in"=w494) -> ("error out"=w501:errorcluster, "Refnum out"=w503:T43)  [unwired: 7 in, 1 out]
        n167 = Unbundle By Name(w482) -> ("Analog Data.Yokogawa.MW100"=w481:refnum<visa-resource-name>, "Power.Yokogawa.WT210.Power VISA Yokogawa WT210"=w480:refnum<visa-resource-name>)
        n168 = control-ref of="Tank Display"() -> (w497:refnum<vi>)
        n169 = call "HEWH Gather Test Data.vi"("MW100"=w481, "Core HEWH Data Station A"=w492, "GEA2?"=FALSE, 3:TRUE ("Update Tank Display"), "Yokogawa WT210"=w480, "error in (no error)"=w501, 11:w497) -> ("Core HEWH Data Station A"=w500:T29, "MW100 Full Data"=w488:string[][], "error out"=w498:errorcluster)  [unwired: 8 in, 2 out]
        n170 = Unbundle By Name(w500) -> ("Draw Count"=w485:i32, "HEWH Specific DAQ.HEWH Data"=→"DAQ Data":T24)
        n171 = Number To Decimal String(number=w485) -> (decimal integer string=w486:string)  [unwired: 1 in]
        n172 = Build Array("Draw Count", w486) -> (w484:string[])
        n173 = Build Array (concatenate)(w489, w488, w484) -> (w483:string[][])
        n174 = Bundle By Name(cluster=w491, "Total Array"=w483) -> (w490:T50)
        n175 = call "UTILITY Release Semaphore.vi"("error in (no error)"=w498, "Refnum in"=w503) -> ("error out"=w493:errorcluster)  [unwired: 9 in]
        n176 = call <vilib>:"Add State(s) to Queue__jki_lib_state_machine.vi"("State(s) in (\"\")"=w505) -> ("States Out"=w504:string)  [unwired: 14 in]
      }
      frame "Check Newfi" {
        n177 = Unbundle By Name(w518) -> ("Total Array"=w522:string[][])
        n178 = call "GEA2 HEWH Appliance Data.vi"("Retry Count"="Retry Count", "Disable ERD A"="Disable ERD A", "error in (no error)"=w512, "Disable Electronic Mixing Valve (EMV) List"="Use EMV List", "GEA2 Event Registration In"=w507, ".NET Refnum in"=w508) -> ("error out"=w511:errorcluster, "HEWH Appliance Data"=w510:string[][], ".NET Refnum out"=w506:refnum<k24>, "Power Display"=→"Set Status":T22)  [unwired: 2 out]
        n179 = call "UTILITY Add Newfi Data To List.vi"("Use Default Headers Main"=TRUE, "Error In"=w511, "Standard GEA2"=w510, "Total Array"=w522) -> ("Error Out"=w521:errorcluster, "Data"=→"MW100 Data":string[][], "Save Data"=w516:string[][])  [unwired: 4 in, 1 out]
        n180 = Bundle By Name(cluster=w518, "Save Data"=w516) -> (w517:T50)
        n181 = call <vilib>:"Add State(s) to Queue__jki_lib_state_machine.vi"("State(s) in (\"\")"=w524) -> ("States Out"=w523:string)  [unwired: 14 in]
      }
      frame "Show Data" {
        n182 = Unbundle By Name(w539) -> ("Plot Array"=w532:dbl[][], "Save Data"=w533:string[][], "Filepath Output.New Summary Created"=w526:bool)
        n183 = call "UTILITY MultiPlot.vi"("Y-Axis-2"="Y-Axis-2", "Y-Axis-1"="Y-Axis-1", "X-Axis"="X-Axis", "Save Data"=w533, "Plot Array"=w532) -> ("Plot Cluster"=w534:T23)  [unwired: 5 in, 1 out]
        n184 = call "UTILITY Create Plot Array.vi"("Save Data"=w533, "Plot Array in"=w532) -> ("Plot Array out"=w531:dbl[][])  [unwired: 8 in, 1 out]
        n185 = case shown="False" "Pause Graph" {
          tunnel: w534 -> [w545 _]
          frame False {
            "XY Graph" <- w545
          }
          frame True {
          }
        }
        n186 = Or(x="Clear Graph Data", y=w526) -> (x .or. y?=w535:bool)
        n187 = case shown="False" w535 {
          tunnel: w531 -> [w543 _]
          tunnel: [w543 dbl[][] [] ("Plot Array out")] -> w530
          frame False {
          }
          frame True {
          }
        }
        n188 = Bundle By Name(cluster=w539, "Plot Array"=w530) -> (w538:T50)
        n189 = call <vilib>:"Add State(s) to Queue__jki_lib_state_machine.vi"("State(s) in (\"\")"=w542) -> ("States Out"=w541:string)  [unwired: 14 in]
      }
      frame "Check Condition" {
        n190 = case shown="\"Time Delay (Seconds)\"" "Cycle Condition" {
          tunnel: [w553 w564] -> w547
          frame "Full Cutout", Default {
            # "Full Cutout"
            n191 = for {
              N: 3 -> [_]
              tunnel: [w557] -> w553
              n192 = local read "Set Status"() -> (w558:T22)
              n193 = Wait Until Next ms Multiple(millisecond multiple=u32 1000) -> ()  [unwired: 1 out]
              n194 = call "HEWH Full Cutout Check.vi"("POWER"=w558) -> ("Heat Source ON (1=ON)"=w560:bool)  [unwired: 8 in, 2 out]
              n195 = Not(x=w560) -> (.not. x?=w557:bool)
            }
            n196 = call "UTILITY Boolean Notifier.vi"("Status"=UTILITY_Notifier."Set", "Set Status"=w553, "name (unnamed)"="Full Cutout") -> ()  [unwired: 7 in, 2 out]
          }
          frame "Time Delay (Seconds)" {
            n197 = local read "Timer Reset"() -> (w563:bool)
            n198 = call "HEWH Trigger Draw Based On Time.vi"("Draw Delay"="Delay Between\nDraws (seconds)", "Timer Reset"=w563) -> ("Trigger Draw"=w564:bool, "Elapsed Time (sec)"=→"Delay Between Draws":dbl)  [unwired: 7 in, 1 out]
          }
        }
        "Start Draw" <- w547
        n199 = call <vilib>:"Add State(s) to Queue__jki_lib_state_machine.vi"("State(s) in (\"\")"=w552) -> ("States Out"=w551:string)  [unwired: 14 in]
      }
      frame "Save Data" {
        n200 = Unbundle By Name(w575) -> ("Filepath Output.Data File Paths.Data File Path"=w570:path, "Washer Controls.Initialize.Washer In.Appliance Details.File Name Output Array"=w571:string[][], "Washer Controls.Initialize.Washer In.Appliance Details.Calibration Output Array"=w572:string[][], "Save Data"=w573:string[][])
        n201 = call "Save File General Data.vi"("Data File Path In"=w570, "File Name Output Array"=w571, "Calibration Output Array"=w572, "Save Data"=w573, "Error In"=w569) -> ("Data File Path Out"=w566:path, "New File"=w567:bool, "Error Out"=w568:errorcluster)  [unwired: 8 in]
        n202 = Bundle By Name(cluster=w575, "Filepath Output.Data File Paths.Data File Path"=w566, "Filepath Output.New Summary Created"=w567) -> (w574:T50)
        n203 = call <vilib>:"Add State(s) to Queue__jki_lib_state_machine.vi"("State(s) in (\"\")"=w577) -> ("States Out"=w576:string)  [unwired: 14 in]
      }
    }
    n204 = case shown="True" "Debug" {
      tunnel: w37 -> [w49 w52]
      tunnel: [w49 w51] -> w35
      tunnel: w36 -> [_ w50]
      frame False {
      }
      frame True {
        n205 = Build Array (concatenate)(w52, w50) -> (w51:string[])
        "States" <- w51
      }
    }
    "JKI Loop" <- w33
  }
  n206 = while {
    tunnel: w7 -> [w589]
    tunnel: [w588] -> w14
    tunnel: w21 -> [w587]
    shift-right: [w585] -> _
    shift-left: _ -> [w586]
    tunnel: w15 -> [w579]
    tunnel: [w578] -> w12
    i -> [w580]
    stop <- w581 stop-if-true
    n207 = local read "Start Draw"() -> (w583:bool)
    n208 = Wait Until Next ms Multiple(millisecond multiple=u32 100) -> ()  [unwired: 1 out]
    n209 = Or(x=w583, y="Start Draw Override") -> (x .or. y?=w582:bool)
    n210 = case shown="True" w582 {
      tunnel: w589 -> [w593 w606]
      tunnel: [w593 w603] -> w588
      tunnel: w587 -> [_ w610]
      tunnel: w586 -> [w592 w609]
      tunnel: [w592 w594] -> w585
      tunnel: w579 -> [w591 w599]
      tunnel: [w591 w596] -> w578
      frame False {
      }
      frame True {
        n211 = flat-sequence {
          tunnel: w606 -> [w634]
          tunnel: [w634] -> w605
          frame #0 {
            n212 = local write "Draw Complete"(FALSE ("Draw Complete")) -> ()
          }
        }
        n213 = Bundle By Name(cluster=w609, "Condition Cluster Output"="Condition Cluster Output") -> (w607:T29)
        n214 = local read "MW100"() -> (w600:refnum<visa-resource-name>)
        n215 = call "HEWH Purge Draw Sequence.vi"("MW100"=w600, "Purge Time (Seconds)"="Purge Time (Seconds)", "Station Draw Info"="Temperature", "Current Cond"="GPM Target", 4:"Gallon Target", "Error In"=w605, "Skip Purge"="Skip Purge", "Core HEWH Data Input"=w607, "Skip Draw"="Skip Draw", "MW100 Sema"=w610) -> ("Core HEWH Data out"=w594:T29, "Error Out"=w604:errorcluster)  [unwired: 8 in]
        n216 = flat-sequence {
          tunnel: w604 -> [w619]
          tunnel: [w619] -> w595
          tunnel: w594 -> [w617]
          tunnel: [w623] -> w602
          tunnel: w599 -> [w621]
          tunnel: [w620] -> w598
          tunnel: w595 -> [w624]
          tunnel: w602 -> [w629]
          tunnel: [w628] -> w601
          tunnel: w598 -> [w626]
          tunnel: [w626] -> w597
          tunnel: [w632] -> w603
          tunnel: w601 -> [w632]
          tunnel: [w630] -> w596
          tunnel: w597 -> [w630]
          frame #0 {
            n217 = Unbundle By Name(w617) -> ("Draw Count"=→"Draw Count":i32)
            "Core HEWH Data out" <- w617
          }
          frame #1 {
            w625 = TRUE ("Draw Start")
            n218 = Generate User Event(user event=w621, event data cluster=w625, error in=w624) -> (user event out=w620:refnum<user-event>, error out=w623:errorcluster)  [unwired: 1 in]
            "Draw Complete" <- w625
            "Timer Reset" <- TRUE ("Draw Start")
          }
          frame #2 {
            n219 = call "UTILITY Delay mS.vi"("Error In"=w629, "milliseconds to wait"=u32 1000) -> ("Error Out"=w628:errorcluster)  [unwired: 13 in]
          }
          frame #3 {
            n220 = local write "Timer Reset"(FALSE ("Draw Start")) -> ()
          }
        }
      }
    }
    n221 = local read "Shutdown"() -> (w581:bool)
    "Draw Loop" <- w580
  }
  n222 = while {
    i -> [w635]
    stop <- w636 stop-if-true
    n223 = Wait Until Next ms Multiple(millisecond multiple=u32 100) -> ()  [unwired: 1 out]
    n224 = call "UTILITY String Notifier.vi"("Status"=UTILITY_Notifier."Read", "name (unnamed)"="Message") -> ("latest notification"=w642:string)  [unwired: 8 in, 1 out]
    n225 = local read "Shutdown"() -> (w638:bool)
    n226 = local write "Message"(w642) -> ()
    n227 = call "UTILITY Boolean Notifier.vi"("Status"=UTILITY_Notifier."Read", "name (unnamed)"="Start UI Loop") -> ("latest READ notification"=w637:bool)  [unwired: 8 in, 1 out]
    n228 = Or(x=w637, y=w638) -> (x .or. y?=w636:bool)
    "Numeric" <- w635
  }
  n229 = call "GEA2 Stop.vi"("GEA2 Reference Out"=w1, "Error In"=w3) -> ("Error Out"=w2:errorcluster)  [unwired: 13 in]
  n230 = Destroy User Event(user event=w12, error in=w14) -> (error out=w13:errorcluster)
  n231 = Merge Errors(w2, w13) -> (→"Error Out":errorcluster)
